vi "Main Scratch Module.vi"(8 "error in (no error)":errorcluster, 11 "main ref":T1) -> (0 "error out":errorcluster)   [LabVIEW 2025]
uses:
  controls/LAB-IQ UI Data.ctl
  Traction Loop/Traction Receipe Enum.ctl
  Scratch Main Enum.ctl
  HEAVE vi's/Heave Write enum.ctl
  b016255a-5e45-488d-a19e-9ca17f1d2554.vi
  230b88c4-d326-49ea-ab42-a573b91a982d.vi
  e59e0919-8fad-4c7c-b2ce-8f9a2e4ae2bd.vi
panel:
  out "Scratch Start Recording":bool
  out "Multi Pass Count":dbl
  out "Multi Scratch with offset":bool
  out "Distance Moved unload":dbl
  out "PID Unload Temp":bool
  out "Scratch Backward Temp":bool
  out "Distance Moved Backward":dbl
  out "Distance Moved":dbl
  out "Scratch Forward Temp":bool
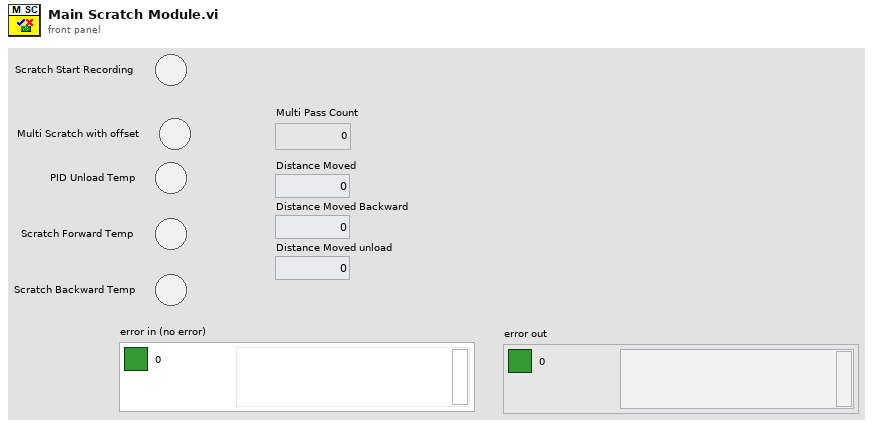
[diagram p1: front panel]
types:
  T1 = typedef "LAB-IQ UI Data.ctl" = cluster{"Main Home Screen":cluster{"GUI":refnum<vi>, "Platform Settings":refnum<vi>, "Configure":refnum<vi>, "Home":refnum<vi>, "EXIT":refnum<vi>, "service 2":refnum<vi>, "MainPage":refnum<vi>, "Analysis":refnum<vi>}, "Platform Settings":cluster{"mm/s  Surge":refnum<vi>, "Update Surge Speed":refnum<vi>, "Drive Error":refnum<vi>, "Disable Axis Jog Soft Limits":refnum<vi>, "mm/s  Sway":refnum<vi>, "Sway and Surge COM Status":refnum<vi>, "Heave COM Status":refnum<vi>, "Enable Platform":refnum<vi>, "Surge Forward Main":refnum<vi>, "Sway Right Main":refnum<vi>, "Sway Left Main":refnum<vi>, "Heave Down Main":refnum<vi>, "Heave Up main":refnum<vi>, "Update Sway Speed":refnum<vi>, "Update Heave Speed":refnum<vi>, "mm/s Heave":refnum<vi>, "mm/sec":refnum<vi>, "mm":refnum<vi>, "Surge Backward Main":refnum<vi>}, "Analysis Screen":cluster{"Analysis Home":refnum<vi>, "Surface Analysis":refnum<vi>, "Imaging":refnum<vi>, "Image Analysis":refnum<vi>, "Post Analysis":refnum<vi>}, "Config Screen":cluster{"Select Load Head":refnum<vi>, "Notes :":refnum<vi>, "FILE":refnum<vi>, "Sample ID :":refnum<vi>, "Operator ID :":refnum<vi>, "Operator Name :":refnum<vi>, "Auto":refnum<vi>}, "Motion Module":cluster{"zNL":refnum<vi>, "NL disp":refnum<vi>, "Rotary Tab":refnum<vi>, "Motion Direction:  3":refnum<vi>, "E.Velocity 2":refnum<vi>, "e.v/ssr 2":refnum<vi>, "Enter Fixed E.Velocity 2":refnum<vi>, "Enter Final SRR 2":refnum<vi>, "Enter initial SRR 2":refnum<vi>, "Enter Fixed SRR 2":refnum<vi>, "Enter the Final E.Velocity (m/s) 2":refnum<vi>, "Enter initial E.Velocity (m/s) 2":refnum<vi>, "Final Speed (RPM) 3":refnum<vi>, "Initial Speed (RPM) 2":refnum<vi>, "Enter the Final Velocity (m/s) 3":refnum<vi>, "Enter initial Velocity (m/s)  3":refnum<vi>, "Ramp Up 2":refnum<vi>, "TEST SELECTION":refnum<vi>, "SPEED SELECTION : ":refnum<vi>, "Angular Oscillation Set":refnum<vi>, "Traction":refnum<vi>, "Step Speed":refnum<vi>, "StepTable For Load-Speed":refnum<vi>, "StepTable For Speed":refnum<vi>, "Surge Forward MM":refnum<vi>, "Surge Backward MM":refnum<vi>, "M3 Image":refnum<vi>, "String 39":refnum<vi>, "Sway Left MM":refnum<vi>, "Sway Right MM":refnum<vi>, "Disable Axis Jog Soft Limits":refnum<vi>, "mm":refnum<vi>, "Heave Down MM":refnum<vi>, "Heave Up MM":refnum<vi>, "Wear Track Diameter (mm)":refnum<vi>, "Set WTD":refnum<vi>, "HomeScratch":refnum<vi>, "HomeRot":refnum<vi>, "PlaceModule":refnum<vi>, "Enter the Angle (Deg)":refnum<vi>, "Enter the Frequency (Hz)":refnum<vi>, "Motion Mode:":refnum<vi>, "LR Sway":refnum<vi>, "Rot Hor":refnum<vi>, "Scratch":refnum<vi>, "LR Cam":refnum<vi>, "MMBack":refnum<vi>, "MMNext":refnum<vi>, "Rot Ver":refnum<vi>, "Rotary Module Selection":refnum<vi>, "calculate rotary":refnum<vi>, "SPEED SELECTION : rotary":refnum<vi>, "Import 2":refnum<vi>, "Save 2":refnum<vi>, "File Path :  2":refnum<vi>, "String 45":refnum<vi>, "StepTable For Speed 3":refnum<vi>, "Enter the Speed(mm/sec)":refnum<vi>, "Enter the Speed(RPM)":refnum<vi>, "Enter Scratch Speed (mm/s):":refnum<vi>, "SwaySpeed Set":refnum<vi>, "Scartch Offset":refnum<vi>, "Motion type:":refnum<vi>, "HomeScratch 2":refnum<vi>, "Enter Scratch length (mm):":refnum<vi>, "Wear Track Diameter":refnum<vi>, "Rotary Speed Exced":refnum<vi>, "Scratch Mode":refnum<vi>, "No of Scratch":refnum<vi>}, "Environmental control":cluster{"Humidity  Status  3":refnum<vi>, "Low Temp  Status  2":refnum<vi>, "TK4 status 2":refnum<vi>, "Stage Temperature":refnum<vi>, "Sample Temperature":refnum<vi>, "Humidity (Amb)":refnum<vi>, "Clear List":refnum<vi>, "Add to list":refnum<vi>, "Wear":refnum<vi>, "Vibration":refnum<vi>, "Humidity (Chamber)":refnum<vi>, "Temperature (Chamber)":refnum<vi>, "ECR ":refnum<vi>, "Temperature (Amb)":refnum<vi>, "Microphone":refnum<vi>, "Acoustic Emission 3":refnum<vi>, "SNext":refnum<vi>, "APBack":refnum<vi>, "Enter the Temperature (°C):":refnum<vi>, "Enter the Stage \nTemperature (°C):":refnum<vi>, "Enter the Humidity (%Rh):":refnum<vi>, "Low Temp":refnum<vi>, "High Temp":refnum<vi>, "Humidity":refnum<vi>, "Sensors Picked":refnum<vi>}, "About Screen":cluster{"Password":refnum<vi>, "Home Service":refnum<vi>, "Advanced Setting":refnum<vi>, "About Tab":refnum<vi>, "ECR Port:":refnum<vi>, "Ramp Port:":refnum<vi>, "Installation/Replacement completed":refnum<vi>, "Loahead":refnum<vi>, "Heave and Surge COM Port:":refnum<vi>, "Sway COM Port:":refnum<vi>, "Temp Modbus:":refnum<vi>, "Humidity Port:":refnum<vi>, "Edit Gain Constants":refnum<vi>, "Save Gain Constants":refnum<vi>}, "Main Screen":cluster{"Main Screen Tab":refnum<vi>, "Angle and Frequency":refnum<vi>, "Stroke (mm)":refnum<vi>, "Angle (Deg)":refnum<vi>, "Main Speed Tab":refnum<vi>, "MTM MOTOR DISPLAY":refnum<vi>, "Disc Speed (m/sec)":refnum<vi>, "Ball Speed (m/sec)":refnum<vi>, "Disc Speed (RPM)":refnum<vi>, "Ball Speed (RPM)":refnum<vi>, "SPEED TAB":refnum<vi>, "Speed (m/sec)":refnum<vi>, "Set Speed (m/sec)":refnum<vi>, "Speed (RPM)":refnum<vi>, "Set Speed":refnum<vi>, "Time Tab":refnum<vi>, "Time ( HH:MM:SS ) 2":refnum<vi>, "Test Duration":refnum<vi>, "Test Duration 4":refnum<vi>, "TEST CYCLE":refnum<vi>, "TOTAL CYCLES":refnum<vi>, "Set Load (N)":refnum<vi>, "Temp Tabs":refnum<vi>, "Heater":refnum<vi>, "TK4 status":refnum<vi>, "ChamberTemp":refnum<vi>, "SetTmp":refnum<vi>, "Controller  Status":refnum<vi>, "ChamberTemp 2":refnum<vi>, "SetTmp 2":refnum<vi>, "Controller  Status 2":refnum<vi>, "ChamberTemp 3":refnum<vi>, "SetTmp 3":refnum<vi>, "Cooling":refnum<vi>, "Load Communication":refnum<vi>, "Ambient \nTemperature":refnum<vi>, "HumCOMStatus":refnum<vi>, "Ambient\n Humidity":refnum<vi>, "Freq (Hz)":refnum<vi>, "Load En":refnum<vi>, "NLt":refnum<vi>, "zNL 2":refnum<vi>, "Humidity On":refnum<vi>, "humidity disp":refnum<vi>, "Set Humidity":refnum<vi>, "NL disp 2":refnum<vi>, "Humidity On 2":refnum<vi>, "humidity disp 2":refnum<vi>, "Set Humidity 2":refnum<vi>, "NL disp 3":refnum<vi>, "AppLoadSeq scratch":refnum<vi>, "Stop Scratch":refnum<vi>, "ClrLog":refnum<vi>, "Trip Log":refnum<vi>, "STOP":refnum<vi>, "Start Test":refnum<vi>, "Test status":refnum<vi>, "AR Led":refnum<vi>, "Data":refnum<vi>, "Health":refnum<vi>, "Sway COM Status":refnum<vi>, "Heave COM Status":refnum<vi>, "Grp Tab":refnum<vi>, "Sub Graph":refnum<vi>, "SD (mm)":refnum<vi>, "Siliding distance Reset Graph":refnum<vi>, "SDGp":refnum<vi>, "Humidity Reset Graph":refnum<vi>, "HumrGp":refnum<vi>, "Acoustic Emission (mV)":refnum<vi>, "Aqucostic Reset Graph":refnum<vi>, "gACQUOS":refnum<vi>, "ECR RESET":refnum<vi>, "ECR":refnum<vi>, "Temperature Reset":refnum<vi>, "Acoustic Emission (mV) 2":refnum<vi>, "Aqucostic Reset Graph 2":refnum<vi>, "gACQUOS 2":refnum<vi>, "ECR RESET 2":refnum<vi>, "ECR 2":refnum<vi>, "Temperature Reset 2":refnum<vi>, "Temperature (deg c)":refnum<vi>, "Speed Reset Graph":refnum<vi>, "Speed Tab":refnum<vi>, "MTM DISC  SPEED":refnum<vi>, "MTM BALL SPEED":refnum<vi>, "speed mm/sec":refnum<vi>, "Hymidity":refnum<vi>, "Humidity Disable trip":refnum<vi>, "CoF Trip  2":refnum<vi>, "Depth Trip":refnum<vi>, "Weart Deapth":refnum<vi>, "Depth Reset Graph":refnum<vi>, "Weart":refnum<vi>, "Depthz":refnum<vi>, "Depth (µm)":refnum<vi>, "WearGp":refnum<vi>, "NL Trip 2":refnum<vi>, "Load pid":refnum<vi>, "Load Disable Trip":refnum<vi>, "Load Reset Graph":refnum<vi>, "NL Display 4":refnum<vi>, "Main Chart 3":refnum<vi>, "BACK":refnum<vi>, "Depth Trip 2":refnum<vi>, "COF TRIP ":refnum<vi>, "Friction Force (N)":refnum<vi>, "FF Reset Graph":refnum<vi>, "FF Disable Trip":refnum<vi>, "FF TRIP":refnum<vi>, "COF Disable Trip":refnum<vi>, "COF Reset Graph":refnum<vi>, "Start Test Temp":refnum<vi>, "zFF":refnum<vi>, "Friction Force (N) Graph":refnum<vi>, "Coefficient of Friction":refnum<vi>, "Scratch Start Test":refnum<vi>, "FF Tab":refnum<vi>, "Cyclic Friction Force (N)":refnum<vi>, "CZ FF":refnum<vi>, "Cyclic Friction Force (N) Graph":refnum<vi>, "Cyclic Coefficient of Friction":refnum<vi>, "Cyclic FF TRIP":refnum<vi>, "Cyclic FF Disable Trip":refnum<vi>, "cyclic COF Disable Trip":refnum<vi>, "cyclic COF TRIP":refnum<vi>, "cyclic COF Reset Graph":refnum<vi>, "Cyclic FF Reset Graph":refnum<vi>, "Test Trip":refnum<vi>, "Multi Scratch Pass":refnum<vi>, "Scratch Start Recording":refnum<vi>}, "Loading":cluster{"Indentation":refnum<vi>, "Reference Sample":refnum<vi>, "Load Cell Communication Slide":refnum<vi>, "com 3":refnum<vi>, "com":refnum<vi>, "DecaForce COM Status":refnum<vi>, "Update":refnum<vi>, "Clear 3":refnum<vi>, "seq":refnum<vi>, "Stribeck table":refnum<vi>, "Stribeck Table  For loading":refnum<vi>, "Loading Mode":refnum<vi>, "Enter the Final Load (N)":refnum<vi>, "Enter the CoF Trip":refnum<vi>, "Enter the Friction Force Trip":refnum<vi>, "Enter the Normal load Trip":refnum<vi>, "Enter the Load  (N)":refnum<vi>, "KiloForce":refnum<vi>, "DecaForce ":refnum<vi>, "MicroForce":refnum<vi>, "LHBack":refnum<vi>, "LHNext":refnum<vi>, "Enter the Loading Rate (N/min)":refnum<vi>, "Message":refnum<vi>, "Warning 2":refnum<vi>, "SSP 0.75":refnum<vi>, "SSP 0.5":refnum<vi>, "SSP 0.3":refnum<vi>, "Warning":refnum<vi>, "gui GIF":refnum<vi>, "Communication is established":refnum<vi>, "AppLoad 4":refnum<vi>, "Multipoint":refnum<vi>, "Load Selection":refnum<vi>}, "PID":cluster{"Ramp MulFac":refnum<vi>, "pulses LoadDiffRamp(2..10)":refnum<vi>, "PulseControlRamp(diff<=3N)":refnum<vi>, "SetLoadDeadband(%) Load(0-10N)":refnum<vi>, "PID gains out delay (microForce)":refnum<vi>, "Ramp":refnum<vi>, "Gain 2":refnum<vi>, "pulses LoadDiff(2..10)":refnum<vi>, "pulses LoadDiff(11..50)":refnum<vi>, "PulseControl(diff<=3N)":refnum<vi>, "SetLoadDeadband(%)  2":refnum<vi>, "Dummy Run":refnum<vi>, "Vertical load (N)":refnum<vi>, "AutoTune":refnum<vi>, "Offset 3 ":refnum<vi>, "apply load":refnum<vi>, "Offset  3":refnum<vi>, "apply load 2":refnum<vi>, "Enter ByPass Load":refnum<vi>, "reinit 3":refnum<vi>, "output range delay":refnum<vi>, "PID gains out delay":refnum<vi>, "Bypass Load":refnum<vi>, "pulsesSent":refnum<vi>, "pulses ":refnum<vi>, "actpid":refnum<vi>, "gFF Rot":refnum<vi>, "pulses LoadDiff(21..1000)":refnum<vi>, "Delay":refnum<vi>, "deadband":refnum<vi>}, "Config Parameters":cluster{"Tab Control 3":refnum<vi>, "Tab Control 19":refnum<vi>, "SAMPLES":refnum<vi>, "Re-initilaize":refnum<vi>, "Filter ON/OFF":refnum<vi>, "TracHomeSurgeOffsetCounts 10MM":refnum<vi>, "TracHomeSwayOffsetCounts 10MM":refnum<vi>, "Acoustic Emission:":refnum<vi>, "Apply Filter (FF)":refnum<vi>, "Filter% 2":refnum<vi>, "Apply Filter (Load)":refnum<vi>, "Filter% ":refnum<vi>, "Sway distance (mm)":refnum<vi>, "Surge distance (mm)":refnum<vi>, "DataSavingLoopDelay(ms)":refnum<vi>, "SAVE 2":refnum<vi>, "Enter Distance":refnum<vi>, "Sway Counts:":refnum<vi>, "Distance (mm): 3":refnum<vi>, "Surge Counts:":refnum<vi>, "Distance (mm): 2":refnum<vi>, "Distance (mm):":refnum<vi>, "Heave Counts:":refnum<vi>, "LRMHomeSurgeOffsetCounts":refnum<vi>, "LRMHomeSwayOffsetCounts":refnum<vi>, "TracHomeSurgeOffsetCounts 20MM":refnum<vi>, "TracHomeSwayOffsetCounts 20MM":refnum<vi>, "RotHomeSwayOffsetCounts":refnum<vi>, "RotHomeSurgeOffsetCounts":refnum<vi>, "Heave distance":refnum<vi>, "Zmm":refnum<vi>, "Heave Pulses/mm":refnum<vi>, "Surge Pulses/mm":refnum<vi>, "Sway Pulses/mm":refnum<vi>, "Heave Pitch":refnum<vi>, "Surge Pitch":refnum<vi>, "Sway Pitch":refnum<vi>, "Heave PPR":refnum<vi>, "Surge PPR":refnum<vi>, "Sway PPR":refnum<vi>, "Tab Control 5":refnum<vi>, "Tab Control 14":refnum<vi>, "Tab Control 26":refnum<vi>, "AE":refnum<vi>, "Heave Loop Delay":refnum<vi>, "Heave PID Speed":refnum<vi>, "Surge Jog Speed":refnum<vi>, "Heave Jog Speed":refnum<vi>, "Sway Loop Delay":refnum<vi>, "Sway PID Speed":refnum<vi>, "Sway Jog Speed":refnum<vi>, "DEPTH TRIP VALUE":refnum<vi>, "LOAD TRIP VALUE":refnum<vi>, "DEPTH TRIP   ENABLE":refnum<vi>, "LOAD TRIP  ENABLE":refnum<vi>, "CYCLIC FF TRIP VALUE":refnum<vi>, "FF TRIP VALUE":refnum<vi>, "CYCLIC CoF TRIP VALUE":refnum<vi>, "COF TRIP VALUE":refnum<vi>, "CYCLIC COF TRIP  ENABLE":refnum<vi>, "CYCLIC FF TRIP  ENABLE":refnum<vi>, "FF TRIP  ENABLE":refnum<vi>, "COF TRIP  ENABLE":refnum<vi>, "JOG TRIP LOAD VALUE (N)":refnum<vi>, "Rotary Vertical":refnum<vi>, "Traction":refnum<vi>, "Scratch":refnum<vi>, "LRM CAM":refnum<vi>, "Sway LRM":refnum<vi>, "Rotary Horizontal":refnum<vi>}, "Loading Com Port":cluster{"ClearAll":refnum<vi>, "Mz(Nm)":refnum<vi>, "My(Nm)":refnum<vi>, "Mx(Nm)":refnum<vi>, "Save Dwell":refnum<vi>, "Acq Delay (ms)":refnum<vi>, "Burst Delay (ms)":refnum<vi>, "model":refnum<vi>, "SN":refnum<vi>, "FFx(N)":refnum<vi>, "Sensor IP":refnum<vi>, "Port":refnum<vi>, "FFy(N)":refnum<vi>, "Load(N)":refnum<vi>, "delete Handle":refnum<vi>, "Create Handle":refnum<vi>, "ft_data":refnum<vi>, "ft_range":refnum<vi>, "ft_data 2":refnum<vi>, "stop 6":refnum<vi>, "running_flag":refnum<vi>, "ft_udp_handle":refnum<vi>, "get-data-return":refnum<vi>, "get-range-return":refnum<vi>, "zero-return":refnum<vi>, "filter-return":refnum<vi>, "initial-return":refnum<vi>, "deleteHandle-result":refnum<vi>, "Load Cell Temp":refnum<vi>, "Load Cell":refnum<vi>, "ZeroAll":refnum<vi>, "FORCE (N)":refnum<vi>, "TORQUE (N-m)":refnum<vi>}, "Heave AND Surge":cluster{"SURGE POSE":refnum<vi>, "error out Read":refnum<vi>, "HEAVE POSE":refnum<vi>, "State":refnum<vi>, "Homed":refnum<vi>, "Sequence ID":refnum<vi>, "error out Write":refnum<vi>, "faultCode":refnum<vi>, "Ack ID":refnum<vi>, "SPEED":refnum<vi>, "Distance":refnum<vi>, "Mode Command":refnum<vi>, "Heave and Surge Read":refnum<vi>, "Read Heave Temp":refnum<vi>, "Spare 15":refnum<vi>, "Spare 14":refnum<vi>, "Spare 13":refnum<vi>, "Spare 12":refnum<vi>, "Spare 11":refnum<vi>, "Spare 10":refnum<vi>, "Spare 9":refnum<vi>, "Spare 8":refnum<vi>, "Spare 7":refnum<vi>, "Spare 6":refnum<vi>, "Spare 5":refnum<vi>, "Spare 4":refnum<vi>, "Spare 2":refnum<vi>, "Spare 1":refnum<vi>, "Node Id":refnum<vi>, "Spare 3":refnum<vi>, "SPARE 4":refnum<vi>, "SPARE 3":refnum<vi>, "SPARE 2":refnum<vi>, "SPARE 1":refnum<vi>, "fwMajor":refnum<vi>, "fwMinor":refnum<vi>, "Manual Write":refnum<vi>, "Heave and Surge Write":refnum<vi>, "SPARE 5":refnum<vi>, "Reserved ":refnum<vi>, "SPARE 8":refnum<vi>, "SPARE 6":refnum<vi>, "SPARE 7":refnum<vi>, "SPARE 17":refnum<vi>, "SPARE 16":refnum<vi>, "SPARE 15":refnum<vi>, "SPARE 14":refnum<vi>, "SPARE 13":refnum<vi>, "SPARE 12":refnum<vi>, "SPARE 11":refnum<vi>, "SPARE 10":refnum<vi>, "SPARE 9":refnum<vi>, "System UPTIME":refnum<vi>, "Missed Packets":refnum<vi>, "faultCode Surge Right":refnum<vi>, "faultCode Surge Left":refnum<vi>, "faultCode Heave":refnum<vi>, "UPLINK HEAVE":refnum<vi>, "DOWNLINK HEAVE":refnum<vi>}, "New PID LOGIC":cluster{"Fine Tune Zone":refnum<vi>, "PID SDelay":refnum<vi>, "Max_pos_limit":refnum<vi>, "Min_pos_limit":refnum<vi>, "i_limit":refnum<vi>, "pct_scale":refnum<vi>, "Deadband":refnum<vi>, "Kd":refnum<vi>, "Ki":refnum<vi>, "Kp":refnum<vi>, "Current Position":refnum<vi>, "Set Load":refnum<vi>, "Current Load":refnum<vi>, "Pulse delta":refnum<vi>, "Init Step":refnum<vi>, "Max Step Linit":refnum<vi>, "min_deadband_floor":refnum<vi>, "dynamic_spindle_noise_scalar":refnum<vi>, "min_finetune_floor":refnum<vi>, "filter_alpha":refnum<vi>, "PID":refnum<vi>}, "SWAY ":cluster{"fwMajor":refnum<vi>, "Homed":refnum<vi>, "Rotary POSE":refnum<vi>, "State":refnum<vi>, "SWAY POSE":refnum<vi>, "Ack ID":refnum<vi>, "faultCode":refnum<vi>, "Node Id":refnum<vi>, "fwMinor":refnum<vi>, "Spare 6":refnum<vi>, "Spare 5":refnum<vi>, "Spare 4":refnum<vi>, "Spare 3":refnum<vi>, "Spare 2":refnum<vi>, "Spare 1":refnum<vi>, "Spare 7":refnum<vi>, "SPARE  5":refnum<vi>, "error out Write  SWAY ":refnum<vi>, "error out Read SWAY ":refnum<vi>, "Manual Write SWAY ":refnum<vi>, "SWAY WRITE":refnum<vi>, "SPARE  4":refnum<vi>, "SPARE  3":refnum<vi>, "SPARE 2":refnum<vi>, "SPARE 1":refnum<vi>, "Spare 15":refnum<vi>, "Spare 14":refnum<vi>, "Spare 13":refnum<vi>, "Spare 12":refnum<vi>, "Spare 11":refnum<vi>, "Spare 9":refnum<vi>, "Spare 8":refnum<vi>, "SPEED":refnum<vi>, "Distance":refnum<vi>, "Mode Command":refnum<vi>, "Sequence ID":refnum<vi>, "SWAY READ":refnum<vi>, "Spare 10":refnum<vi>, "Read SWAY Temp":refnum<vi>, "faultCode Sway ":refnum<vi>, "Missed Packets":refnum<vi>, "System UPTIME sway":refnum<vi>, "SPARE 6":refnum<vi>, "SPARE 7":refnum<vi>, "SPARE 9":refnum<vi>, "SPARE 11":refnum<vi>, "SPARE 10":refnum<vi>, "SPARE 8":refnum<vi>, "SPARE 13":refnum<vi>, "SPARE 12":refnum<vi>, "SPARE 17":refnum<vi>, "SPARE 16":refnum<vi>, "SPARE 15":refnum<vi>, "SPARE 14":refnum<vi>, "Reserved":refnum<vi>, "faultCode Rotary":refnum<vi>, "UPLINK SWAY":refnum<vi>, "DOWNLINK SWAY":refnum<vi>}, "Analysis Screen":cluster{"Analysis Home":refnum<vi>, "Refresh 2":refnum<vi>, "MEAN 4":refnum<vi>, "SD 4":refnum<vi>, "VARIANCE 4":refnum<vi>, "MEAN  3":refnum<vi>, "SD  3":refnum<vi>, "VARIANCE  3":refnum<vi>, "MEAN 2":refnum<vi>, "SD  2":refnum<vi>, "VARIANCE 2":refnum<vi>, "MEAN":refnum<vi>, "SD":refnum<vi>, "VARIANCE":refnum<vi>, "File 4 Discription":refnum<vi>, "OPEN 4":refnum<vi>, "File Name 4":refnum<vi>, "OPEN 3":refnum<vi>, "File 3 Discription":refnum<vi>, "File Name 3":refnum<vi>, "Y-AXIS":refnum<vi>, "X-AXIS":refnum<vi>, "XY Graph":refnum<vi>, "File Name 2":refnum<vi>, "File Name 1":refnum<vi>, "OPEN 2":refnum<vi>, "OPEN 1":refnum<vi>, "File 1 Discription ":refnum<vi>, "File 2 Discription":refnum<vi>, "Export":refnum<vi>, "File Format":refnum<vi>}, "Traction":cluster{"faultCode Traction 2":refnum<vi>, "faultCode Traction 1":refnum<vi>, "Missed Packets":refnum<vi>, "System UPTIME Traction":refnum<vi>, "SPARE 17":refnum<vi>, "SPARE 16":refnum<vi>, "SPARE 15":refnum<vi>, "SPARE 14":refnum<vi>, "SPARE 13":refnum<vi>, "SPARE 12":refnum<vi>, "SPARE 11":refnum<vi>, "SPARE 10":refnum<vi>, "SPARE 9":refnum<vi>, "SPARE 8":refnum<vi>, "SPARE 7":refnum<vi>, "SPARE 6":refnum<vi>, "Reserved":refnum<vi>, "SPARE  5":refnum<vi>, "Manual Write TRACTION":refnum<vi>, "TRACTION WRITE":refnum<vi>, "SPARE  4":refnum<vi>, "SPARE  3":refnum<vi>, "SPARE 2":refnum<vi>, "SPARE 1":refnum<vi>, "Spare 7":refnum<vi>, "Spare 6":refnum<vi>, "Spare 5":refnum<vi>, "Spare 4":refnum<vi>, "Spare 2":refnum<vi>, "Spare 1":refnum<vi>, "Node Id":refnum<vi>, "Read TRACTION Temp":refnum<vi>, "fwMinor":refnum<vi>, "fwMajor":refnum<vi>, "faultCode":refnum<vi>, "TRACTION POSE":refnum<vi>, "TRACTION POSE 2":refnum<vi>, "Homed":refnum<vi>, "State":refnum<vi>, "Ack ID":refnum<vi>, "SPEED":refnum<vi>, "Distance":refnum<vi>, "Mode Command":refnum<vi>, "Sequence ID":refnum<vi>, "error out Read TRACTION":refnum<vi>, "error out Write  TRACTION":refnum<vi>, "TRACTION READ":refnum<vi>, "Spare 3":refnum<vi>, "Downlink traction":refnum<vi>, "Uplink Traction":refnum<vi>}, "Traction reciepe":cluster{"SRR Sweep Range (%) Stribeck":refnum<vi>, "Traction Receipe":refnum<vi>, "Total Execution Time":refnum<vi>, "Total Steps":refnum<vi>, "Duration / Step (s)  Stribeck":refnum<vi>, "STRIBECK Fixed SRR List (%)":refnum<vi>, "Duration / Step (s) Traction":refnum<vi>, "SRR Sweep Range (%) traction":refnum<vi>, "Rolling Speed (mm/s)":refnum<vi>, "Temperature Stages (°C)":refnum<vi>, "Ball Load (N)":refnum<vi>, "Lubricant Name":refnum<vi>, "Profile File Name":refnum<vi>, "SET entrainment Velocity":refnum<vi>, "Test Array Size":refnum<vi>, "SRR INDEX [ STRIBECK]":refnum<vi>, "Stribeck Size":refnum<vi>, "SET SRR":refnum<vi>, "ELAPSED TIMER ":refnum<vi>, "BALL SET RPM":refnum<vi>, "DISC SET RPM":refnum<vi>, "SET LOAD":refnum<vi>, "TEMPERATURE READ":refnum<vi>, "SET TEMPERATURE":refnum<vi>, "Traction Size":refnum<vi>, "DISC SPEED (rpm)":refnum<vi>, "BALL SPEED (rpm)":refnum<vi>, "BALL WEAR TRACK":refnum<vi>, "DISC WEARTRACK":refnum<vi>, "SRR INDEX [ TRACTION]":refnum<vi>, "Start Index Type":refnum<vi>, "Enum - Menu":refnum<vi>, "Ball (mm/sec)":refnum<vi>, "Disc (mm/sec)":refnum<vi>}, "Traction Control":cluster{"HomeTraction":refnum<vi>, "Demo Mode Display":refnum<vi>, "Traction Message":refnum<vi>, "Traction Step Update Details":refnum<vi>, "Main Tab sequence for selection":refnum<vi>, "Ramp Tab":refnum<vi>, "e.v/ssr":refnum<vi>, "Enter Fixed E.Velocity":refnum<vi>, "Enter Final SRR":refnum<vi>, "Enter initial SRR":refnum<vi>, "Enter Fixed SRR":refnum<vi>, "Enter the Final E.Velocity (m/s)":refnum<vi>, "Enter initial E.Velocity (m/s)":refnum<vi>, "Ball WTD":refnum<vi>, "E.Velocity":refnum<vi>, "Enter the Final Velocity (m/s)":refnum<vi>, "Enter initial Velocity (m/s)":refnum<vi>, "Ramp Up   Disc":refnum<vi>, "Initial DiscSpeed (RPM)":refnum<vi>, "Final Speed (RPM) Ball":refnum<vi>, "Final Speed (RPM)":refnum<vi>, "Initial Speed (RPM) Ball":refnum<vi>, "Enter the Final Velocity (m/s) Ball":refnum<vi>, "Enter initial Velocity (m/s) Ball":refnum<vi>, "Ramp Up":refnum<vi>, "ExceedBallSpeed step":refnum<vi>, "ExceedDiscSpeed":refnum<vi>, "BallSpeed Exceed Indication":refnum<vi>, "Apply":refnum<vi>, "SPEED SELECTION : MTM":refnum<vi>, "SPEED SELECTION : MTM 2":refnum<vi>, "TEST SELECTION (MTM)":refnum<vi>, "MTM Test Selection":refnum<vi>, "File Path Tab":refnum<vi>, "File Path String":refnum<vi>, "Save":refnum<vi>, "Save  2":refnum<vi>, "Import ":refnum<vi>, "File Path :":refnum<vi>, "Step Sequence Indication Tab":refnum<vi>, "Step Sequence Indication":refnum<vi>, "Calculate Step":refnum<vi>, "StepTable":refnum<vi>, "ExceedDiscSpeed  Cinstant Speed":refnum<vi>, "ExceedBallSpeed Constant":refnum<vi>, "TEST SELECTION (MTM) 2":refnum<vi>, "SPEED SELECTION : MTM 3":refnum<vi>, "MTM Test Selection 2":refnum<vi>, "Enter the Speed (m/sec): ":refnum<vi>, "Enter the Speed (m/sec):  2":refnum<vi>, "Enter the Speed (RPM):":refnum<vi>, "Lower Spped ":refnum<vi>, "Upper":refnum<vi>, "Enter the Speed (RPM):Ball":refnum<vi>, "Disc Motion Direction: ":refnum<vi>, "Ball Motion Direction :":refnum<vi>, "Motion Mode: ":refnum<vi>, "Wear Track Diameter (mm) ":refnum<vi>, "Disc Speed Indicator":refnum<vi>, "ExceedBallSpeed":refnum<vi>}, "Acquostic":cluster{"Last Config Rejected ":refnum<vi>, "rx command count":refnum<vi>, "Current Filter Id":refnum<vi>, "Isolated Gain":refnum<vi>, "DAQ Status":refnum<vi>, "error out":refnum<vi>, "error in (no error)":refnum<vi>, "Uplink Packet":refnum<vi>, "data out":refnum<vi>, "Downlink Packet":refnum<vi>, "Signal Energy":refnum<vi>, "Amplitude db_AE":refnum<vi>, "Peak Amplitude":refnum<vi>, "AE Ring-Down Counts":refnum<vi>, "Gains":refnum<vi>, "Manual Write Acquostic":refnum<vi>}}
  T2 = enum32{"Setup", "Load Head", "Motion Module", "Environment", "Begin"}
  T3 = typedef "Scratch Main Enum.ctl" = enum16{"Init", "Start", "Load", "Scratch Forward", "Scratch Backward", "Unload", "Offest", "Close"}
  T4 = typedef "Heave Write enum.ctl" = enum16{"INIT", "WRITE", "CLOSE", "REINIT"}
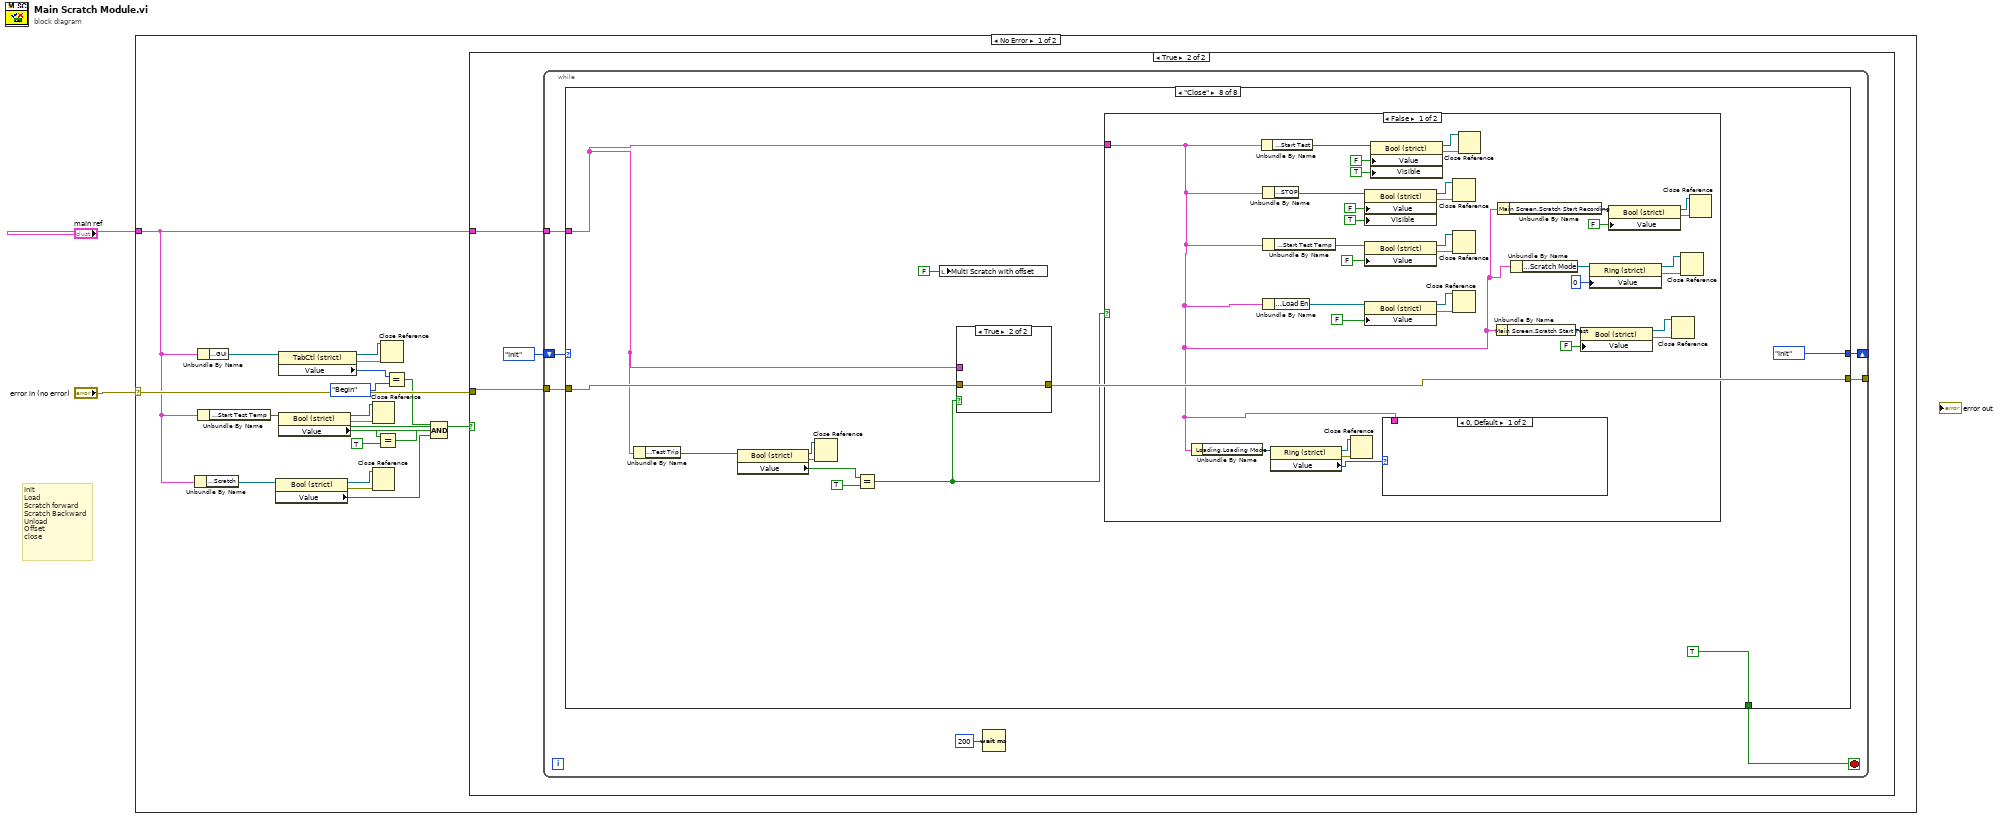
[diagram p0: block diagram]
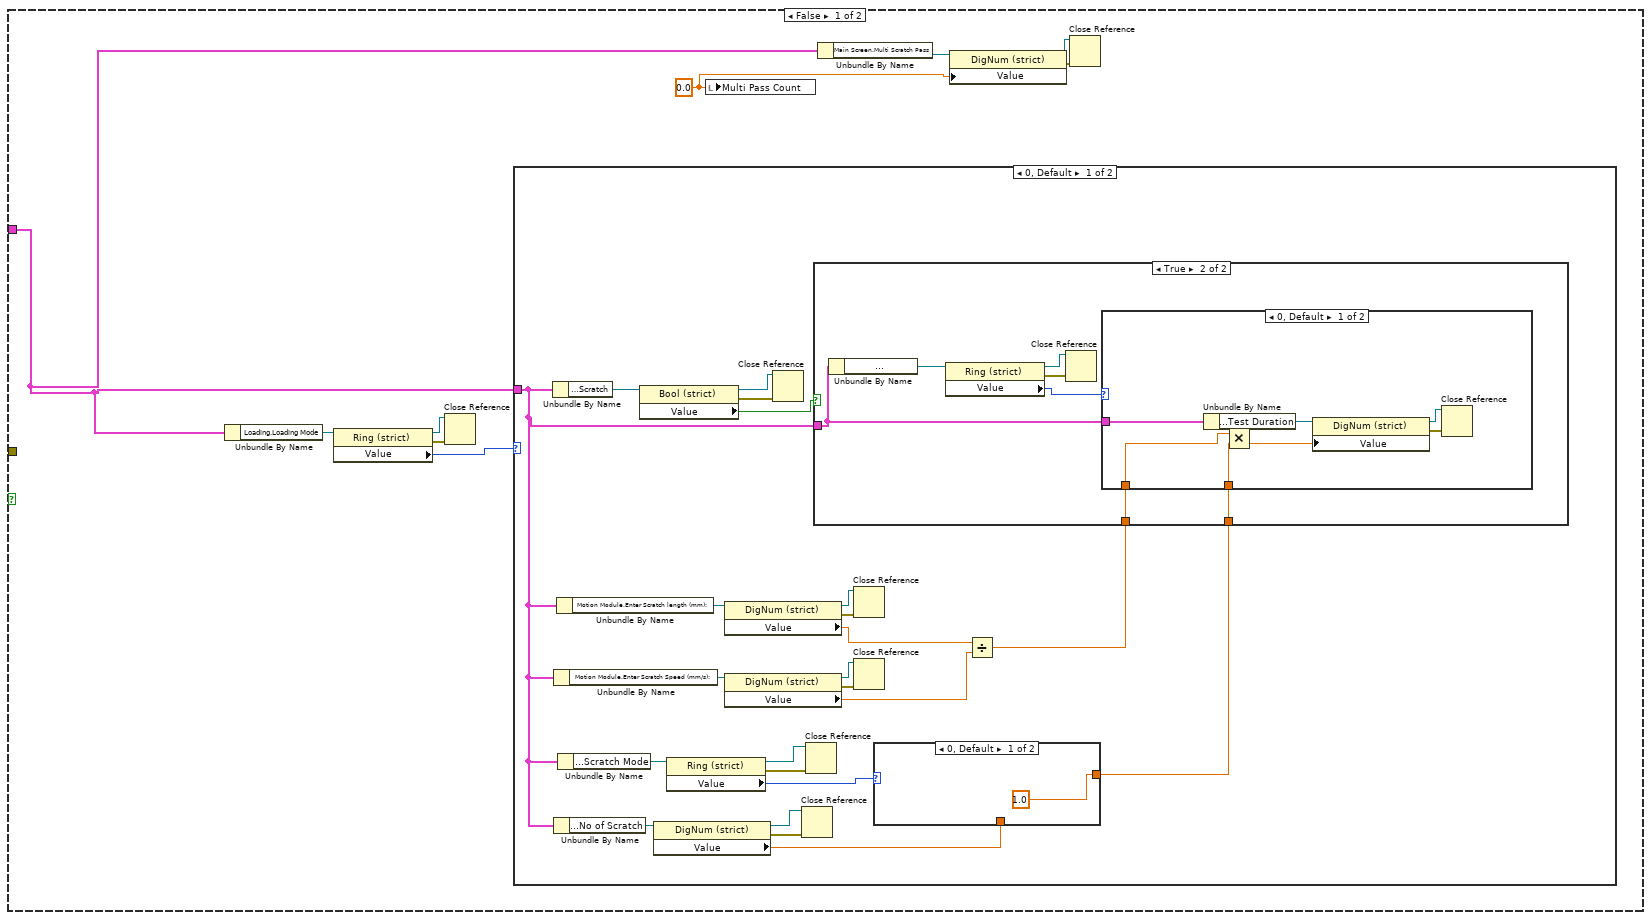
[diagram p2: hidden frame]
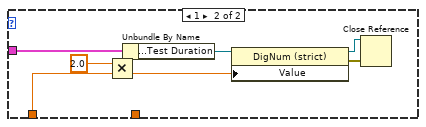
[diagram p5: hidden frame]
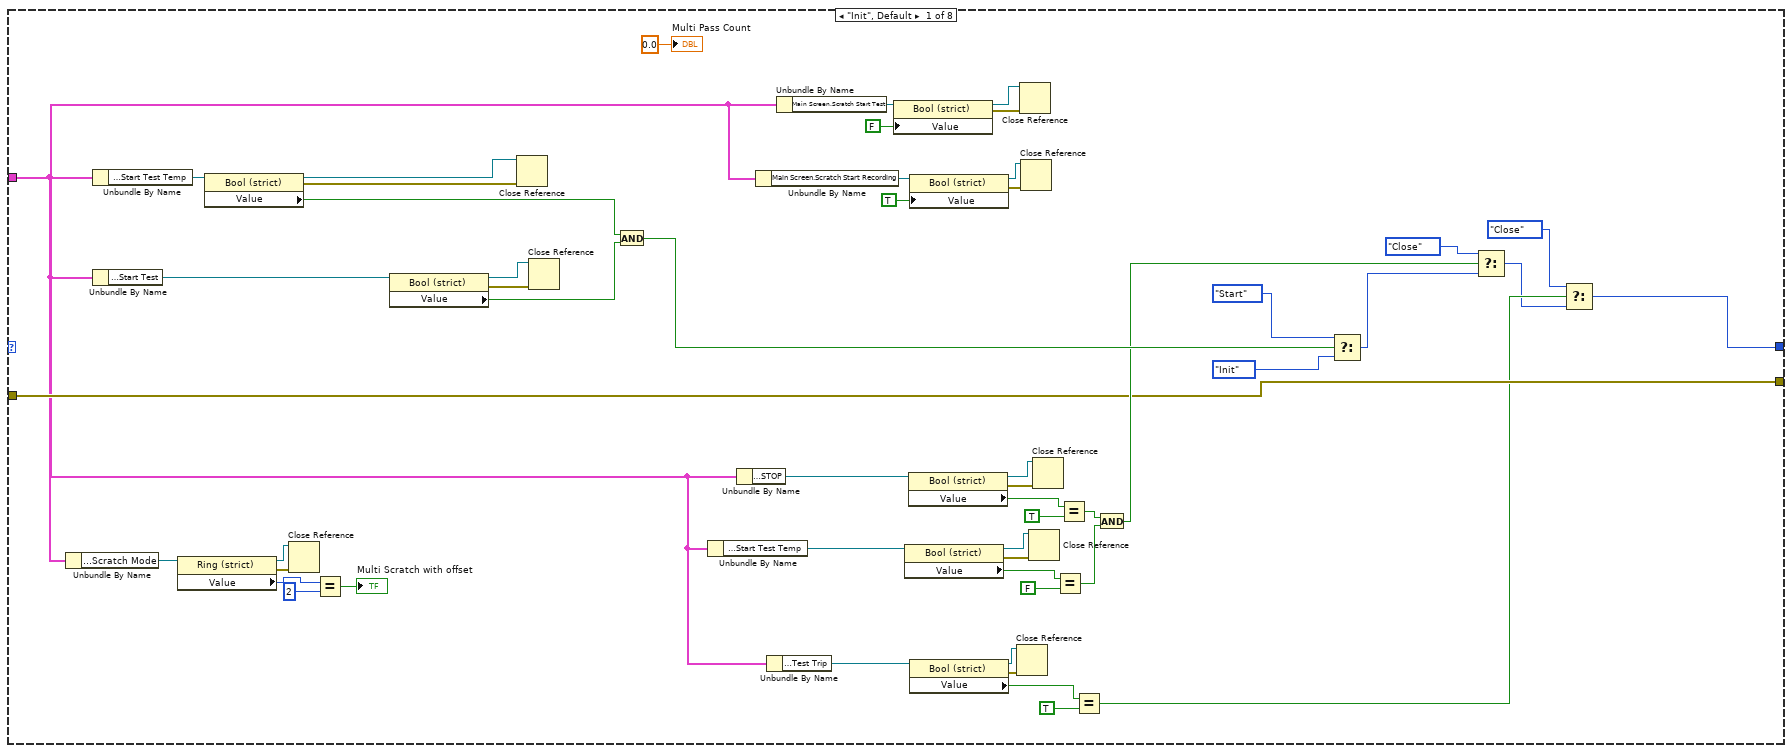
[diagram p7: hidden frame]
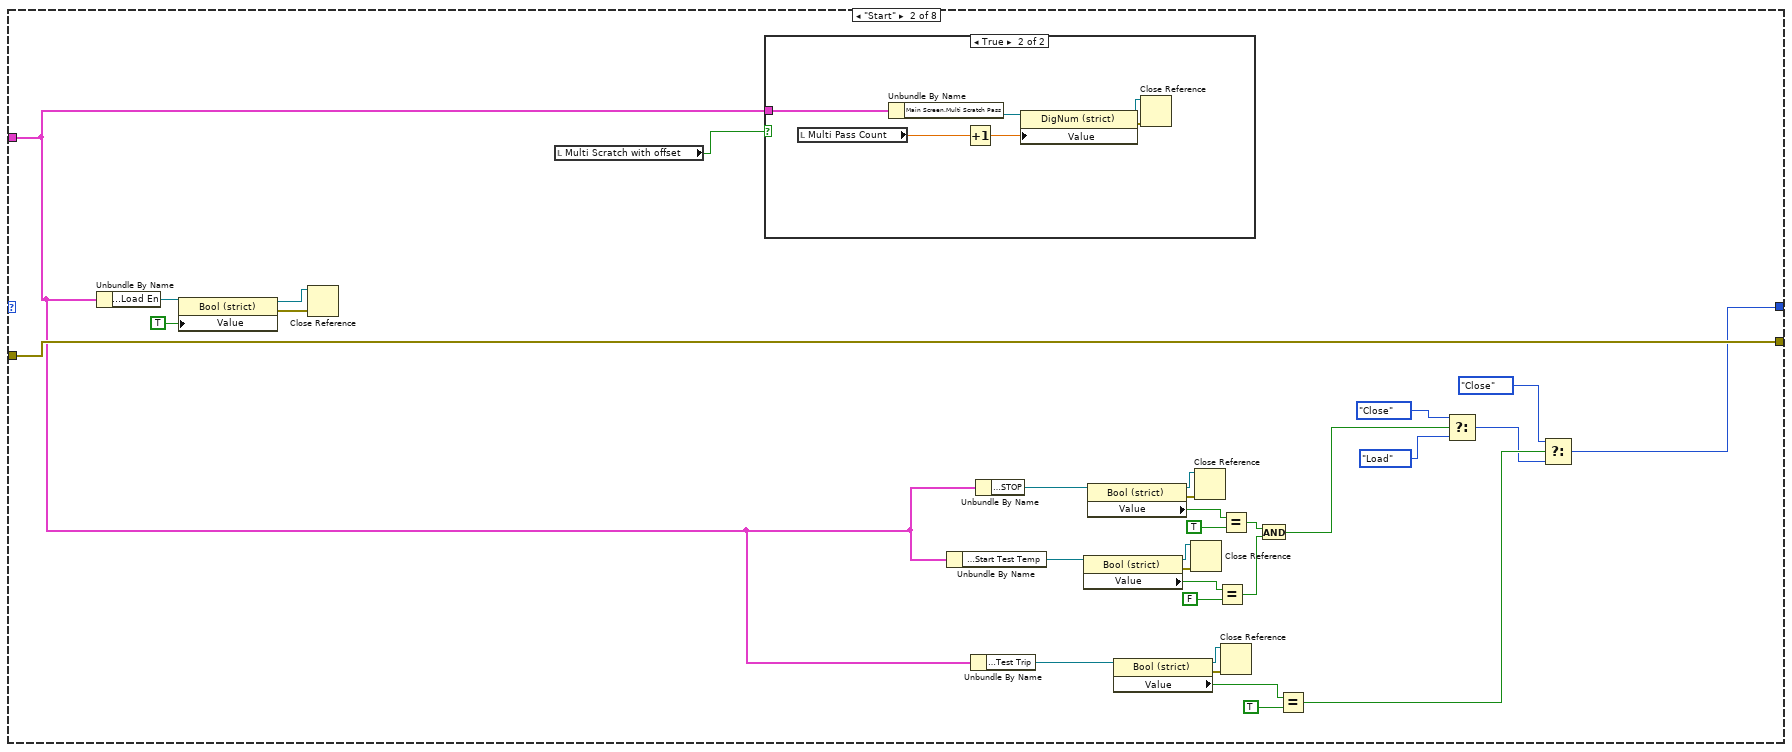
[diagram p8: hidden frame]
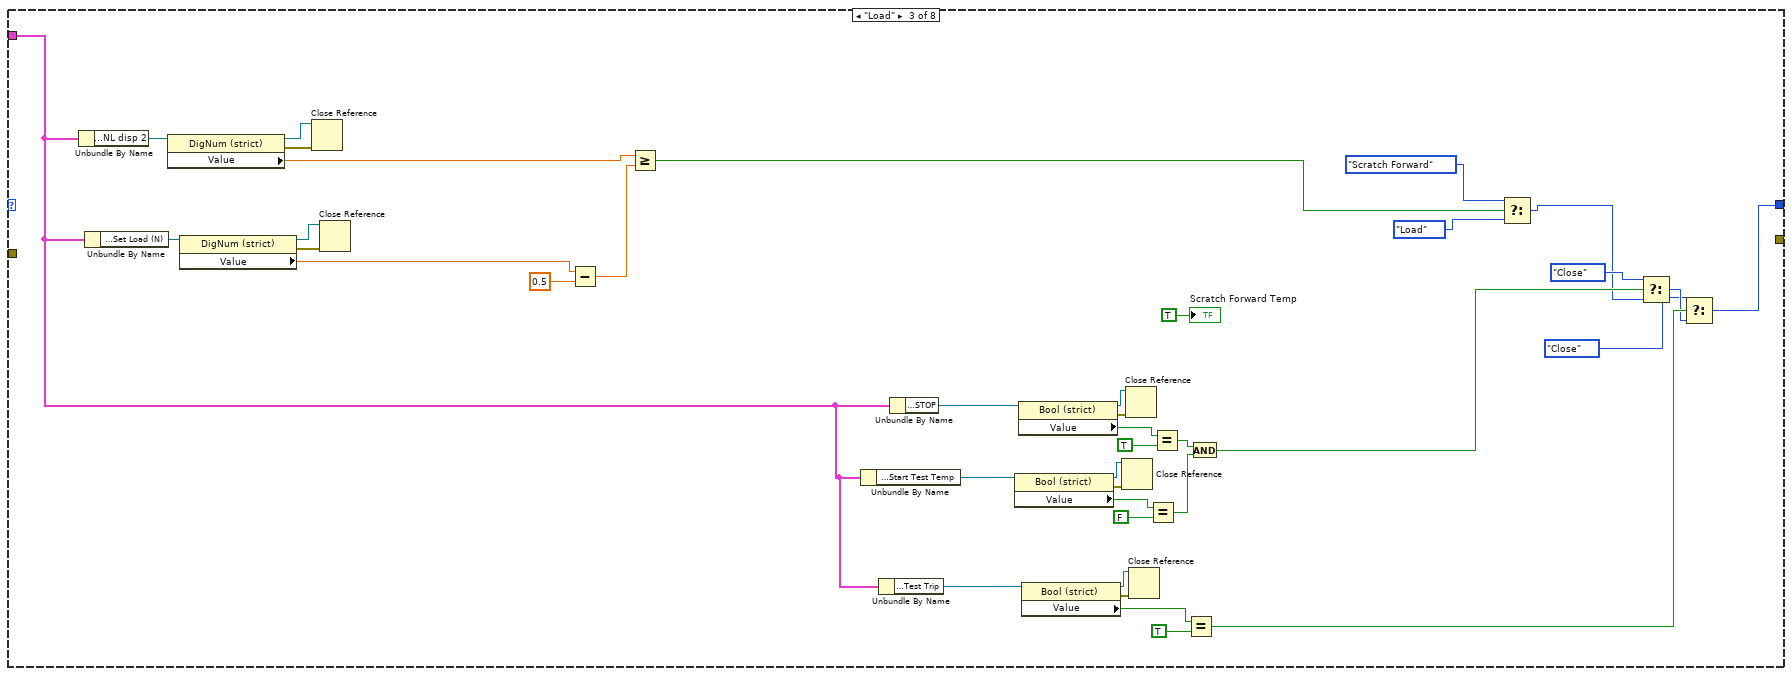
[diagram p10: hidden frame]
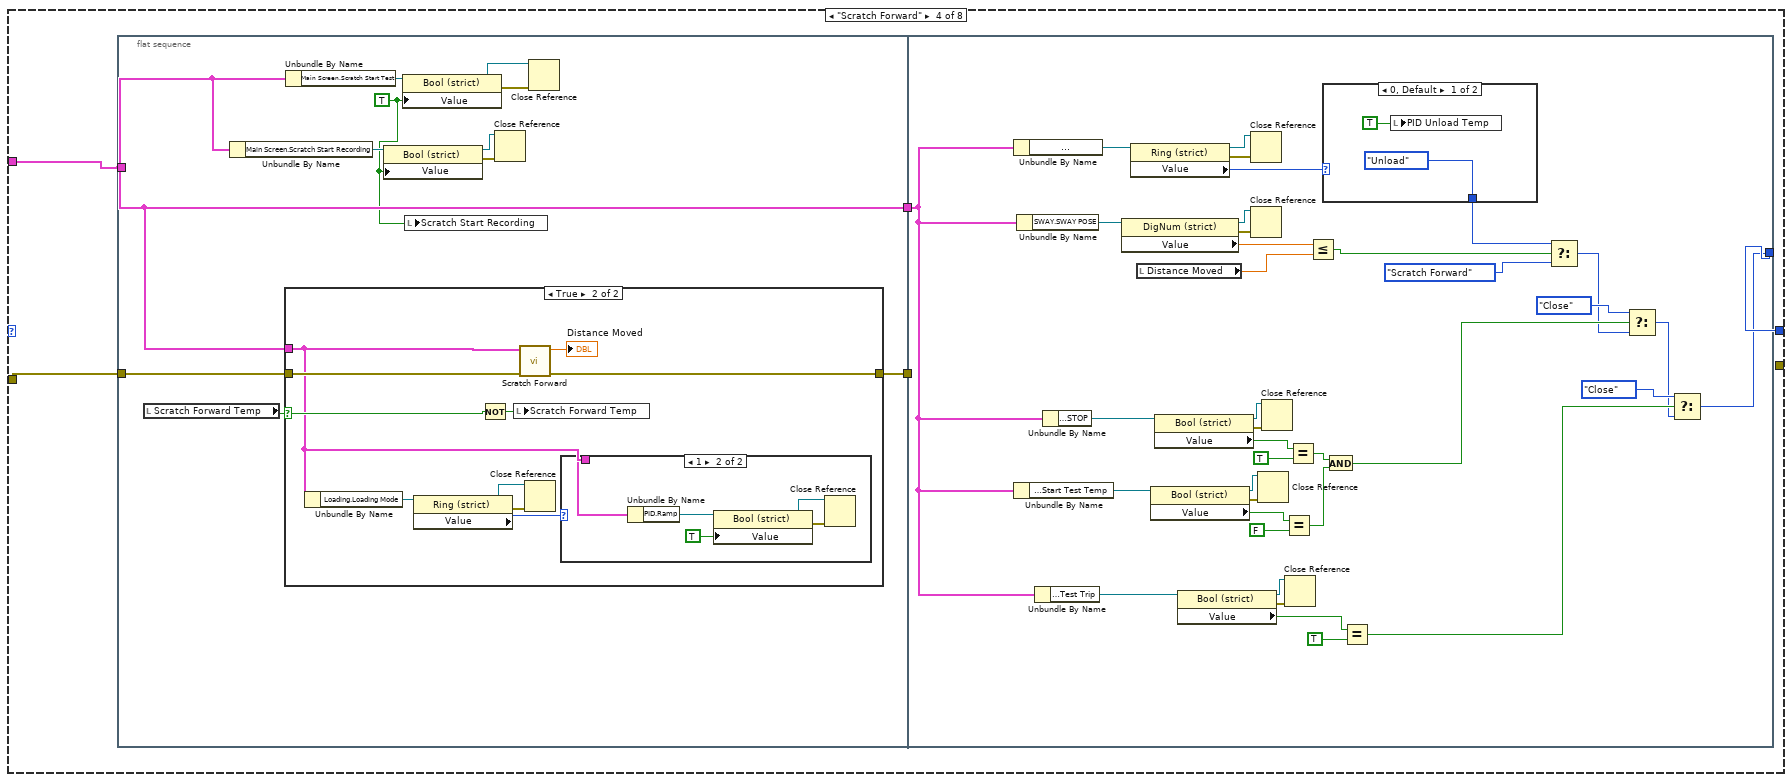
[diagram p11: hidden frame]
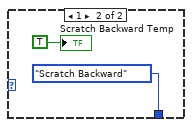
[diagram p14: hidden frame]
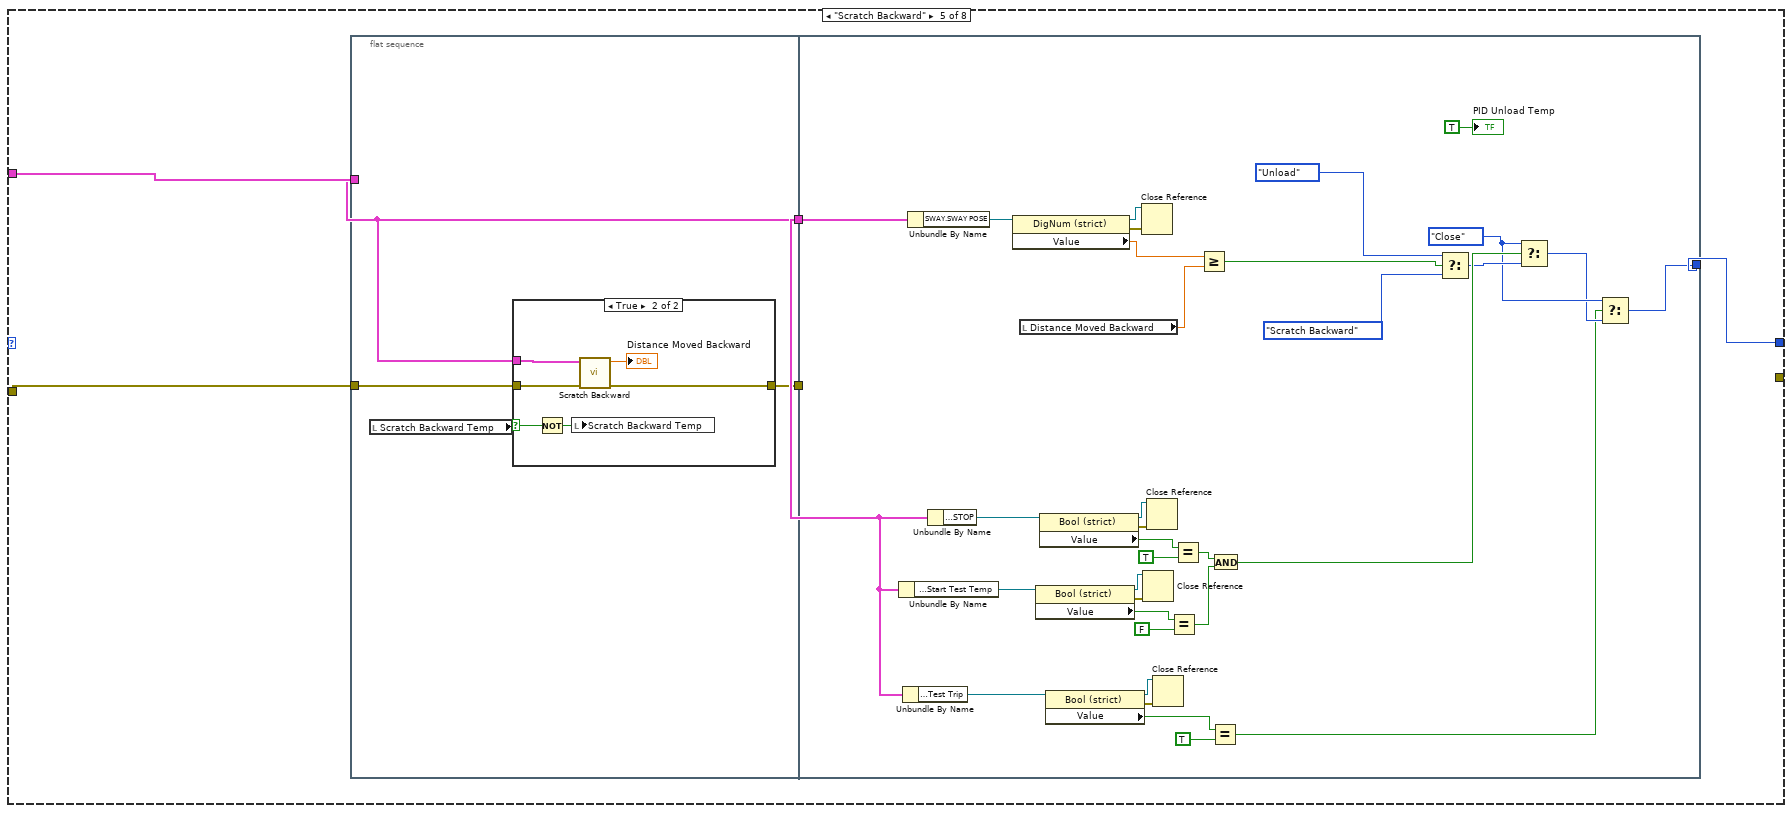
[diagram p15: hidden frame]
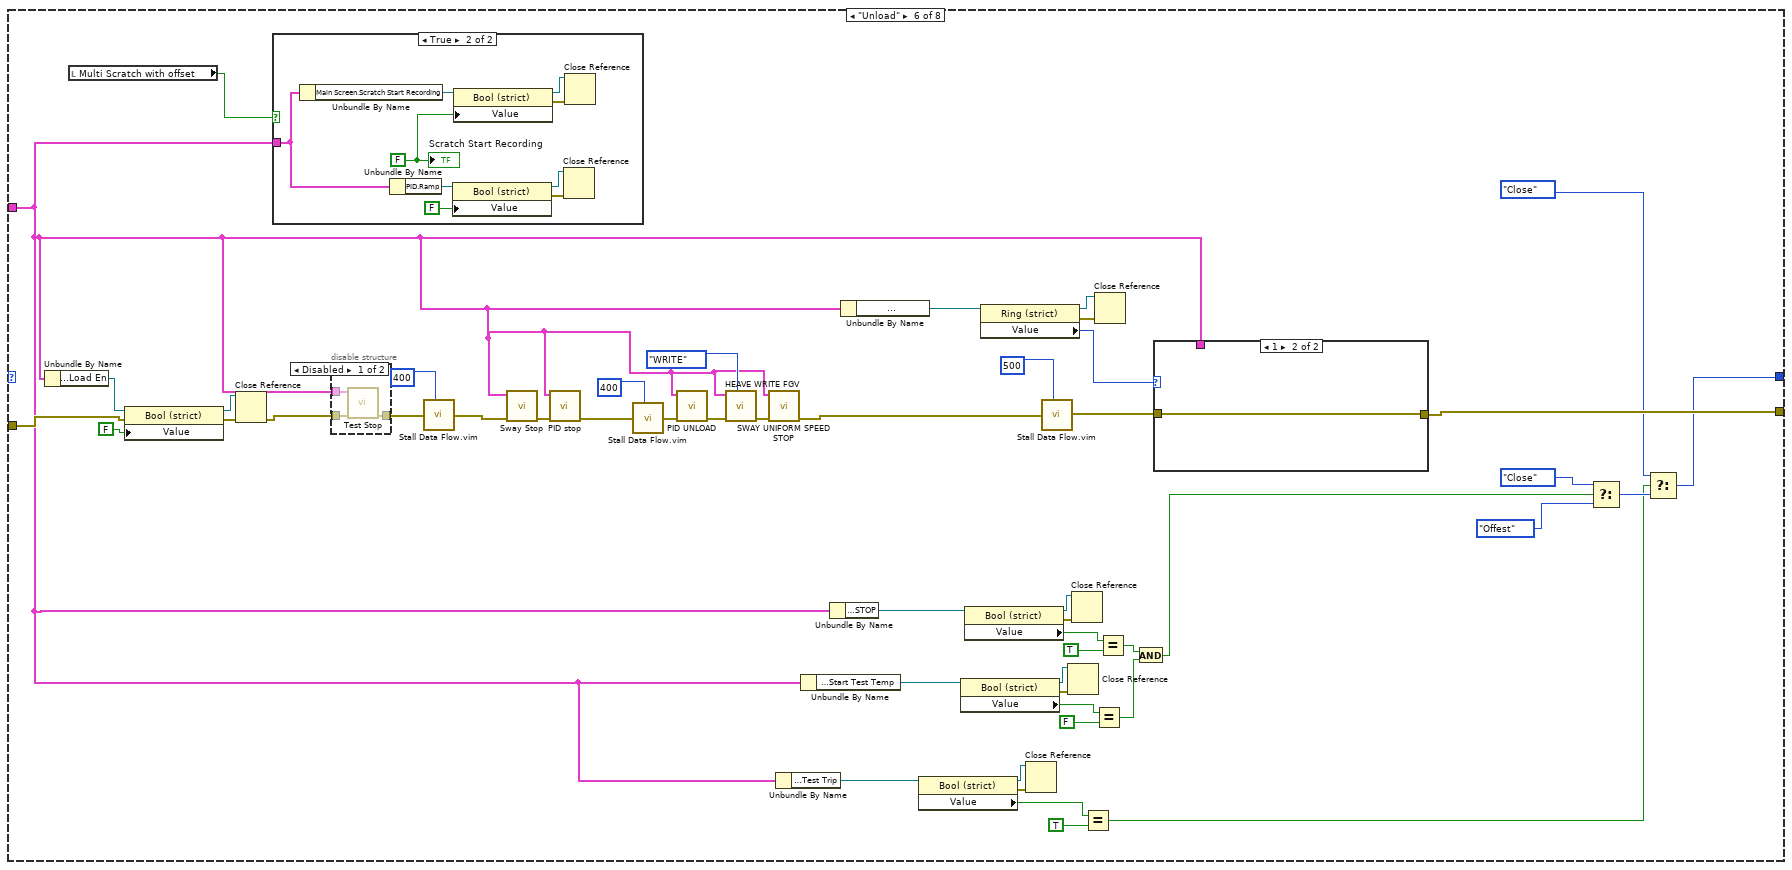
[diagram p17: hidden frame]
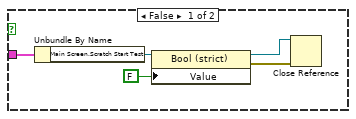
[diagram p18: hidden frame]
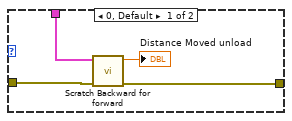
[diagram p20: hidden frame]
diagram:
  # "Init \nLoad\nScratch forward\nScratch Backward\nUnload\nOffset\nclose"
  n1 = case shown="No Error" "error in (no error)" {
    selector: "error in (no error)" -> [w21 _]
    tunnel: "main ref" -> [w4 _]
    frame No Error {
      n2 = Unbundle By Name(w4) -> ("Motion Module.Scratch"=w8:refnum<vi>)
      n3 = Unbundle By Name(w4) -> ("Main Home Screen.GUI"=w18:refnum<vi>)
      n4 = Unbundle By Name(w4) -> ("Main Screen.Start Test Temp"=w13:refnum<vi>)
      n5 = property class="Bool (strict)"(reference=w8) -> (reference out=w5:refnum<vi>, error out=w7:errorcluster, "Value"=w6:bool)  [unwired: 1 in]
      n6 = property class="TabCtl (strict)"(reference=w18) -> (reference out=w20:refnum<vi>, error out=w19:errorcluster, "Value"=w17:T2)  [unwired: 1 in]
      n7 = property class="Bool (strict)"(reference=w13) -> (reference out=w11:refnum<vi>, error out=w12:errorcluster, "Value"=w14:bool)  [unwired: 1 in]
      n8 = Close Reference(reference=w11, error in (no error)=w12) -> ()  [unwired: 1 out]
      n9 = Close Reference(reference=w5, error in (no error)=w7) -> ()  [unwired: 1 out]
      n10 = Equal?(x=w14, y=TRUE) -> (x = y?=w10:bool)
      n11 = Close Reference(reference=w20, error in (no error)=w19) -> ()  [unwired: 1 out]
      n12 = Equal?(x=w17, y=T2."Begin" ("Value")) -> (x = y?=w15:bool)
      n13 = Compound Arithmetic op=AND(w15, w10, w6) -> (w3:bool)
      n14 = case shown="True" w3 {
        tunnel: w4 -> [w23 w78]
        tunnel: w21 -> [_ w77]
        frame False {
          w22 = 0.0 ("Multi Pass Count")
          n15 = Unbundle By Name(w23) -> ("Loading.Loading Mode"=w30:refnum<vi>)
          n16 = property class="Ring (strict)"(reference=w30) -> (reference out=w28:refnum<vi>, error out=w29:errorcluster, "Value"=w27:u16)  [unwired: 1 in]
          n17 = Close Reference(reference=w28, error in (no error)=w29) -> ()  [unwired: 1 out]
          n18 = case shown="0, Default" w27 {
            tunnel: w23 -> [w33 _]
            frame 0, Default {
              n19 = Unbundle By Name(w33) -> ("Motion Module.Scratch"=w51:refnum<vi>)
              n20 = Unbundle By Name(w33) -> ("Motion Module.Enter Scratch Speed (mm/s):"=w46:refnum<vi>)
              n21 = Unbundle By Name(w33) -> ("Motion Module.No of Scratch"=w35:refnum<vi>)
              n22 = Unbundle By Name(w33) -> ("Motion Module.Enter Scratch length (mm):"=w47:refnum<vi>)
              n23 = Unbundle By Name(w33) -> ("Motion Module.Scratch Mode"=w39:refnum<vi>)
              n24 = property class="Bool (strict)"(reference=w51) -> (reference out=w53:refnum<vi>, error out=w52:errorcluster, "Value"=w50:bool)  [unwired: 1 in]
              n25 = property class="DigNum (strict)"(reference=w35) -> (reference out=w34:refnum<vi>, error out=w36:errorcluster, "Value"=w32:dbl)  [unwired: 1 in]
              n26 = property class="Ring (strict)"(reference=w39) -> (reference out=w40:refnum<vi>, error out=w38:errorcluster, "Value"=w37:u16)  [unwired: 1 in]
              n27 = property class="DigNum (strict)"(reference=w47) -> (reference out=w49:refnum<vi>, error out=w48:errorcluster, "Value"=w43:dbl)  [unwired: 1 in]
              n28 = property class="DigNum (strict)"(reference=w46) -> (reference out=w44:refnum<vi>, error out=w45:errorcluster, "Value"=w42:dbl)  [unwired: 1 in]
              n29 = Close Reference(reference=w53, error in (no error)=w52) -> ()  [unwired: 1 out]
              n30 = Close Reference(reference=w34, error in (no error)=w36) -> ()  [unwired: 1 out]
              n31 = Close Reference(reference=w40, error in (no error)=w38) -> ()  [unwired: 1 out]
              n32 = Close Reference(reference=w49, error in (no error)=w48) -> ()  [unwired: 1 out]
              n33 = Close Reference(reference=w44, error in (no error)=w45) -> ()  [unwired: 1 out]
              n34 = case shown="0, Default" w37 {
                tunnel: [1.0 w55] -> w31
                tunnel: w32 -> [_ w55]
                frame 0, Default {
                }
                frame 2 {
                }
              }
              n35 = Divide(x=w43, y=w42) -> (x/y=w41:dbl)
              n36 = case shown="True" w50 {
                tunnel: w33 -> [_ w57]
                tunnel: w41 -> [_ w58]
                tunnel: w31 -> [_ w56]
                frame False {
                }
                frame True {
                  n37 = Unbundle By Name(w57) -> ("Motion Module.Motion type:"=w61:refnum<vi>)
                  n38 = property class="Ring (strict)"(reference=w61) -> (reference out=w62:refnum<vi>, error out=w60:errorcluster, "Value"=w59:u16)  [unwired: 1 in]
                  n39 = Close Reference(reference=w62, error in (no error)=w60) -> ()  [unwired: 1 out]
                  n40 = case shown="0, Default" w59 {
                    tunnel: w58 -> [w64 w72]
                    tunnel: w57 -> [w66 w73]
                    tunnel: w56 -> [w63 _]
                    frame 0, Default {
                      n41 = Unbundle By Name(w66) -> ("Main Screen.Test Duration"=w68:refnum<vi>)
                      n42 = Multiply(x=w64, y=w63) -> (x*y=w65:dbl)
                      n43 = property class="DigNum (strict)"(reference=w68, "Value"=w65) -> (reference out=w69:refnum<vi>, error out=w67:errorcluster)  [unwired: 1 in]
                      n44 = Close Reference(reference=w69, error in (no error)=w67) -> ()  [unwired: 1 out]
                    }
                    frame 1 {
                      n45 = Multiply(x=2.0, y=w72) -> (x*y=w71:dbl)
                      n46 = Unbundle By Name(w73) -> ("Main Screen.Test Duration"=w75:refnum<vi>)
                      n47 = property class="DigNum (strict)"(reference=w75, "Value"=w71) -> (reference out=w76:refnum<vi>, error out=w74:errorcluster)  [unwired: 1 in]
                      n48 = Close Reference(reference=w76, error in (no error)=w74) -> ()  [unwired: 1 out]
                    }
                  }
                }
              }
            }
            frame 1 {
            }
          }
          n49 = local write "Multi Pass Count"(w22) -> ()
          n50 = Unbundle By Name(w23) -> ("Main Screen.Multi Scratch Pass"=w26:refnum<vi>)
          n51 = property class="DigNum (strict)"(reference=w26, "Value"=w22) -> (reference out=w24:refnum<vi>, error out=w25:errorcluster)  [unwired: 1 in]
          n52 = Close Reference(reference=w24, error in (no error)=w25) -> ()  [unwired: 1 out]
        }
        frame True {
          n53 = while {
            shift-right: [w84] -> _
            shift-left: Scratch_Main_Enum."Init" -> [w86]
            tunnel: w78 -> [w85]
            tunnel: w77 -> [w83]
            tunnel: [w81] -> _
            stop <- w80 stop-if-true
            n54 = case shown="\"Close\"" w86 {
              tunnel: w85 -> [w87 w139 w180 w219 w292 w344 w414 w496]
              tunnel: [w99 w141 w176 w215 w288 w338 w418 Scratch_Main_Enum."Init"] -> w84
              tunnel: w83 -> [w112 w165 _ w218 w291 w350 w447 w504]
              tunnel: [w112 w165 _ _ _ w382 w442 w502] -> w81
              tunnel: [_ _ _ _ _ _ _ TRUE] -> w80
              frame "Init", Default {
                n55 = Unbundle By Name(w87) -> ("Motion Module.Scratch Mode"=w97:refnum<vi>)
                n56 = Unbundle By Name(w87) -> ("Main Screen.Start Test Temp"=w135:refnum<vi>)
                n57 = Unbundle By Name(w87) -> ("Main Screen.Start Test"=w132:refnum<vi>)
                n58 = property class="Ring (strict)"(reference=w97) -> (reference out=w98:refnum<vi>, error out=w96:errorcluster, "Value"=w95:u16)  [unwired: 1 in]
                n59 = property class="Bool (strict)"(reference=w135) -> (reference out=w136:refnum<vi>, error out=w134:errorcluster, "Value"=w130:bool)  [unwired: 1 in]
                n60 = Close Reference(reference=w98, error in (no error)=w96) -> ()  [unwired: 1 out]
                n61 = Equal?(x=w95, y=u16 2) -> (x = y?=→"Multi Scratch with offset":bool)
                n62 = property class="Bool (strict)"(reference=w132) -> (reference out=w131:refnum<vi>, error out=w133:errorcluster, "Value"=w129:bool)  [unwired: 1 in]
                n63 = Close Reference(reference=w136, error in (no error)=w134) -> ()  [unwired: 1 out]
                n64 = Close Reference(reference=w131, error in (no error)=w133) -> ()  [unwired: 1 out]
                n65 = And(x=w130, y=w129) -> (x .and. y?=w128:bool)
                n66 = Unbundle By Name(w87) -> ("Main Screen.Start Test Temp"=w122:refnum<vi>)
                n67 = Unbundle By Name(w87) -> ("Main Screen.STOP"=w125:refnum<vi>)
                n68 = Unbundle By Name(w87) -> ("Main Screen.Scratch Start Recording"=w90:refnum<vi>)
                n69 = Unbundle By Name(w87) -> ("Main Screen.Test Trip"=w105:refnum<vi>)
                n70 = Unbundle By Name(w87) -> ("Main Screen.Scratch Start Test"=w110:refnum<vi>)
                n71 = property class="Bool (strict)"(reference=w110, "Value"=FALSE) -> (reference out=w111:refnum<vi>, error out=w109:errorcluster)  [unwired: 1 in]
                n72 = property class="Bool (strict)"(reference=w122) -> (reference out=w120:refnum<vi>, error out=w121:errorcluster, "Value"=w123:bool)  [unwired: 1 in]
                n73 = property class="Bool (strict)"(reference=w125) -> (reference out=w127:refnum<vi>, error out=w126:errorcluster, "Value"=w124:bool)  [unwired: 1 in]
                n74 = property class="Bool (strict)"(reference=w90, "Value"=TRUE) -> (reference out=w91:refnum<vi>, error out=w89:errorcluster)  [unwired: 1 in]
                n75 = property class="Bool (strict)"(reference=w105) -> (reference out=w107:refnum<vi>, error out=w106:errorcluster, "Value"=w103:bool)  [unwired: 1 in]
                n76 = Close Reference(reference=w107, error in (no error)=w106) -> ()  [unwired: 1 out]
                n77 = Close Reference(reference=w111, error in (no error)=w109) -> ()  [unwired: 1 out]
                n78 = Close Reference(reference=w91, error in (no error)=w89) -> ()  [unwired: 1 out]
                n79 = Close Reference(reference=w120, error in (no error)=w121) -> ()  [unwired: 1 out]
                n80 = Close Reference(reference=w127, error in (no error)=w126) -> ()  [unwired: 1 out]
                n81 = Equal?(x=w123, y=FALSE) -> (x = y?=w118:bool)
                n82 = Equal?(x=w124, y=TRUE) -> (x = y?=w119:bool)
                n83 = Equal?(x=w103, y=TRUE) -> (x = y?=w102:bool)
                n84 = And(x=w119, y=w118) -> (x .and. y?=w115:bool)
                n85 = Select(t=Scratch_Main_Enum."Start", s=w128, f=Scratch_Main_Enum."Init") -> (s? t:f=w113:T3)
                n86 = Select(t=Scratch_Main_Enum."Close", s=w115, f=w113) -> (s? t:f=w100:T3)
                n87 = Select(t=Scratch_Main_Enum."Close", s=w102, f=w100) -> (s? t:f=w99:T3)
                "Multi Pass Count" <- 0.0 ("Multi Pass Count")
              }
              frame "Start" {
                n88 = Unbundle By Name(w139) -> ("Main Screen.Load En"=w169:refnum<vi>)
                n89 = property class="Bool (strict)"(reference=w169, "Value"=TRUE) -> (reference out=w167:refnum<vi>, error out=w168:errorcluster)  [unwired: 1 in]
                n90 = Close Reference(reference=w167, error in (no error)=w168) -> ()  [unwired: 1 out]
                n91 = local read "Multi Scratch with offset"() -> (w140:bool)
                n92 = case shown="True" w140 {
                  tunnel: w139 -> [_ w172]
                  frame False {
                  }
                  frame True {
                    n93 = local read "Multi Pass Count"() -> (w171:dbl)
                    n94 = Unbundle By Name(w172) -> ("Main Screen.Multi Scratch Pass"=w175:refnum<vi>)
                    n95 = Increment(x=w171) -> (x+1=w170:dbl)
                    n96 = property class="DigNum (strict)"(reference=w175, "Value"=w170) -> (reference out=w173:refnum<vi>, error out=w174:errorcluster)  [unwired: 1 in]
                    n97 = Close Reference(reference=w173, error in (no error)=w174) -> ()  [unwired: 1 out]
                  }
                }
                n98 = Unbundle By Name(w139) -> ("Main Screen.Start Test Temp"=w159:refnum<vi>)
                n99 = Unbundle By Name(w139) -> ("Main Screen.Test Trip"=w147:refnum<vi>)
                n100 = Unbundle By Name(w139) -> ("Main Screen.STOP"=w162:refnum<vi>)
                n101 = property class="Bool (strict)"(reference=w159) -> (reference out=w157:refnum<vi>, error out=w158:errorcluster, "Value"=w160:bool)  [unwired: 1 in]
                n102 = property class="Bool (strict)"(reference=w162) -> (reference out=w164:refnum<vi>, error out=w163:errorcluster, "Value"=w161:bool)  [unwired: 1 in]
                n103 = property class="Bool (strict)"(reference=w147) -> (reference out=w149:refnum<vi>, error out=w148:errorcluster, "Value"=w145:bool)  [unwired: 1 in]
                n104 = Close Reference(reference=w157, error in (no error)=w158) -> ()  [unwired: 1 out]
                n105 = Close Reference(reference=w164, error in (no error)=w163) -> ()  [unwired: 1 out]
                n106 = Equal?(x=w160, y=FALSE) -> (x = y?=w155:bool)
                n107 = Equal?(x=w161, y=TRUE) -> (x = y?=w156:bool)
                n108 = Close Reference(reference=w149, error in (no error)=w148) -> ()  [unwired: 1 out]
                n109 = And(x=w156, y=w155) -> (x .and. y?=w151:bool)
                n110 = Equal?(x=w145, y=TRUE) -> (x = y?=w143:bool)
                n111 = Select(t=Scratch_Main_Enum."Close", s=w151, f=Scratch_Main_Enum."Load") -> (s? t:f=w142:T3)
                n112 = Select(t=Scratch_Main_Enum."Close", s=w143, f=w142) -> (s? t:f=w141:T3)
              }
              frame "Load" {
                n113 = Unbundle By Name(w180) -> ("Main Screen.NL disp 2"=w214:refnum<vi>)
                n114 = Unbundle By Name(w180) -> ("Main Screen.Set Load (N)"=w210:refnum<vi>)
                n115 = property class="DigNum (strict)"(reference=w214) -> (reference out=w212:refnum<vi>, error out=w213:errorcluster, "Value"=w205:dbl)  [unwired: 1 in]
                n116 = property class="DigNum (strict)"(reference=w210) -> (reference out=w209:refnum<vi>, error out=w211:errorcluster, "Value"=w208:dbl)  [unwired: 1 in]
                n117 = Close Reference(reference=w212, error in (no error)=w213) -> ()  [unwired: 1 out]
                n118 = Close Reference(reference=w209, error in (no error)=w211) -> ()  [unwired: 1 out]
                n119 = Subtract(x=w208, y=0.5) -> (x-y=w206:dbl)
                n120 = Greater Or Equal?(x=w205, y=w206) -> (x >= y?=w202:bool)
                n121 = Unbundle By Name(w180) -> ("Main Screen.Start Test Temp"=w194:refnum<vi>)
                n122 = Unbundle By Name(w180) -> ("Main Screen.Test Trip"=w183:refnum<vi>)
                n123 = Unbundle By Name(w180) -> ("Main Screen.STOP"=w197:refnum<vi>)
                n124 = property class="Bool (strict)"(reference=w194) -> (reference out=w192:refnum<vi>, error out=w193:errorcluster, "Value"=w195:bool)  [unwired: 1 in]
                n125 = property class="Bool (strict)"(reference=w197) -> (reference out=w199:refnum<vi>, error out=w198:errorcluster, "Value"=w196:bool)  [unwired: 1 in]
                n126 = property class="Bool (strict)"(reference=w183) -> (reference out=w185:refnum<vi>, error out=w184:errorcluster, "Value"=w181:bool)  [unwired: 1 in]
                n127 = Close Reference(reference=w192, error in (no error)=w193) -> ()  [unwired: 1 out]
                n128 = Close Reference(reference=w199, error in (no error)=w198) -> ()  [unwired: 1 out]
                n129 = Close Reference(reference=w185, error in (no error)=w184) -> ()  [unwired: 1 out]
                n130 = Equal?(x=w195, y=FALSE) -> (x = y?=w190:bool)
                n131 = Equal?(x=w196, y=TRUE) -> (x = y?=w191:bool)
                n132 = Equal?(x=w181, y=TRUE) -> (x = y?=w179:bool)
                n133 = And(x=w191, y=w190) -> (x .and. y?=w187:bool)
                n134 = Select(t=Scratch_Main_Enum."Scratch Forward", s=w202, f=Scratch_Main_Enum."Load") -> (s? t:f=w186:T3)
                n135 = Select(t=Scratch_Main_Enum."Close", s=w187, f=w186) -> (s? t:f=w178:T3)
                n136 = Select(t=Scratch_Main_Enum."Close", s=w179, f=w178) -> (s? t:f=w176:T3)
                "Scratch Forward Temp" <- TRUE ("Scratch Forward Temp")
              }
              frame "Scratch Forward" {
                n137 = flat-sequence {
                  tunnel: w219 -> [w221]
                  tunnel: w218 -> [w229]
                  tunnel: [w228] -> w217
                  tunnel: [w221] -> w216
                  tunnel: w217 -> [_]
                  tunnel: w216 -> [w251]
                  tunnel: [w247] -> w215
                  frame #0 {
                    w220 = TRUE ("Value")
                    n138 = local read "Scratch Forward Temp"() -> (w230:bool)
                    n139 = Unbundle By Name(w221) -> ("Main Screen.Scratch Start Recording"=w223:refnum<vi>)
                    n140 = case shown="True" w230 {
                      selector: w230 -> [_ w241]
                      tunnel: w221 -> [_ w232]
                      tunnel: w229 -> [w231 w239]
                      tunnel: [w231 w238] -> w228
                      frame False {
                      }
                      frame True {
                        n141 = Unbundle By Name(w232) -> ("Loading.Loading Mode"=w236:refnum<vi>)
                        n142 = property class="Ring (strict)"(reference=w236) -> (reference out=w234:refnum<vi>, error out=w235:errorcluster, "Value"=w233:u16)  [unwired: 1 in]
                        n143 = Not(x=w241) -> (.not. x?=w240:bool)
                        n144 = local write "Scratch Forward Temp"(w240) -> ()
                        n145 = call "Scratch Forward.vi"("error in (no error)"=w239, "main ref"=w232) -> ("error out"=w238:errorcluster, "Distance Moved"=→"Distance Moved":dbl)  [unwired: 8 in]
                        n146 = Close Reference(reference=w234, error in (no error)=w235) -> ()  [unwired: 1 out]
                        n147 = case shown="1" w233 {
                          tunnel: w232 -> [_ w243]
                          frame 0, Default {
                          }
                          frame 1 {
                            n148 = Unbundle By Name(w243) -> ("PID.Ramp"=w244:refnum<vi>)
                            n149 = property class="Bool (strict)"(reference=w244, "Value"=TRUE) -> (reference out=w246:refnum<vi>, error out=w245:errorcluster)  [unwired: 1 in]
                            n150 = Close Reference(reference=w246, error in (no error)=w245) -> ()  [unwired: 1 out]
                          }
                        }
                      }
                    }
                    n151 = Unbundle By Name(w221) -> ("Main Screen.Scratch Start Test"=w226:refnum<vi>)
                    n152 = property class="Bool (strict)"(reference=w223, "Value"=w220) -> (reference out=w224:refnum<vi>, error out=w222:errorcluster)  [unwired: 1 in]
                    n153 = property class="Bool (strict)"(reference=w226, "Value"=w220) -> (reference out=w227:refnum<vi>, error out=w225:errorcluster)  [unwired: 1 in]
                    n154 = local write "Scratch Start Recording"(w220) -> ()
                    n155 = Close Reference(reference=w224, error in (no error)=w222) -> ()  [unwired: 1 out]
                    n156 = Close Reference(reference=w227, error in (no error)=w225) -> ()  [unwired: 1 out]
                  }
                  frame #1 {
                    n157 = Unbundle By Name(w251) -> ("Motion Module.Motion type:"=w276:refnum<vi>)
                    n158 = Unbundle By Name(w251) -> ("Main Screen.Start Test Temp"=w265:refnum<vi>)
                    n159 = Unbundle By Name(w251) -> ("SWAY.SWAY POSE"=w282:refnum<vi>)
                    n160 = Unbundle By Name(w251) -> ("Main Screen.Test Trip"=w254:refnum<vi>)
                    n161 = Unbundle By Name(w251) -> ("Main Screen.STOP"=w268:refnum<vi>)
                    n162 = property class="DigNum (strict)"(reference=w282) -> (reference out=w281:refnum<vi>, error out=w283:errorcluster, "Value"=w280:sgl)  [unwired: 1 in]
                    n163 = property class="Ring (strict)"(reference=w276) -> (reference out=w277:refnum<vi>, error out=w275:errorcluster, "Value"=w274:u16)  [unwired: 1 in]
                    n164 = local read "Distance Moved"() -> (w279:dbl)
                    n165 = property class="Bool (strict)"(reference=w265) -> (reference out=w263:refnum<vi>, error out=w264:errorcluster, "Value"=w266:bool)  [unwired: 1 in]
                    n166 = property class="Bool (strict)"(reference=w268) -> (reference out=w270:refnum<vi>, error out=w269:errorcluster, "Value"=w267:bool)  [unwired: 1 in]
                    n167 = property class="Bool (strict)"(reference=w254) -> (reference out=w256:refnum<vi>, error out=w255:errorcluster, "Value"=w252:bool)  [unwired: 1 in]
                    n168 = Close Reference(reference=w277, error in (no error)=w275) -> ()  [unwired: 1 out]
                    n169 = Close Reference(reference=w281, error in (no error)=w283) -> ()  [unwired: 1 out]
                    n170 = Close Reference(reference=w263, error in (no error)=w264) -> ()  [unwired: 1 out]
                    n171 = Close Reference(reference=w270, error in (no error)=w269) -> ()  [unwired: 1 out]
                    n172 = Equal?(x=w266, y=FALSE) -> (x = y?=w261:bool)
                    n173 = Close Reference(reference=w256, error in (no error)=w255) -> ()  [unwired: 1 out]
                    n174 = Equal?(x=w267, y=TRUE) -> (x = y?=w262:bool)
                    n175 = Less Or Equal?(x=w280, y=w279) -> (x <= y?=w278:bool)
                    n176 = case shown="0, Default" w274 {
                      tunnel: [Scratch_Main_Enum."Unload" Scratch_Main_Enum."Scratch Backward"] -> w273
                      frame 0, Default {
                        n177 = local write "PID Unload Temp"(TRUE ("PID Unload Temp")) -> ()
                      }
                      frame 1 {
                        "Scratch Backward Temp" <- TRUE
                      }
                    }
                    n178 = And(x=w262, y=w261) -> (x .and. y?=w258:bool)
                    n179 = Equal?(x=w252, y=TRUE) -> (x = y?=w249:bool)
                    n180 = Select(t=w273, s=w278, f=Scratch_Main_Enum."Scratch Forward") -> (s? t:f=w257:T3)
                    n181 = Select(t=Scratch_Main_Enum."Close", s=w258, f=w257) -> (s? t:f=w248:T3)
                    n182 = Select(t=Scratch_Main_Enum."Close", s=w249, f=w248) -> (s? t:f=w247:T3)
                  }
                }
              }
              frame "Scratch Backward" {
                n183 = flat-sequence {
                  tunnel: w292 -> [w294]
                  tunnel: w291 -> [w296]
                  tunnel: [w295] -> w290
                  tunnel: [w294] -> w289
                  tunnel: w290 -> [_]
                  tunnel: w289 -> [w308]
                  tunnel: [w305] -> w288
                  frame #0 {
                    n184 = local read "Scratch Backward Temp"() -> (w293:bool)
                    n185 = case shown="True" w293 {
                      selector: w293 -> [_ w299]
                      tunnel: w294 -> [_ w303]
                      tunnel: w296 -> [w297 w302]
                      tunnel: [w297 w301] -> w295
                      frame False {
                      }
                      frame True {
                        n186 = Not(x=w299) -> (.not. x?=w298:bool)
                        n187 = local write "Scratch Backward Temp"(w298) -> ()
                        n188 = call "Scratch Backward.vi"("error in (no error)"=w302, "main ref"=w303) -> ("error out"=w301:errorcluster, "Distance Moved"=→"Distance Moved Backward":dbl)  [unwired: 8 in]
                      }
                    }
                  }
                  frame #1 {
                    w307 = Scratch_Main_Enum."Close"
                    n189 = Unbundle By Name(w308) -> ("Main Screen.Start Test Temp"=w322:refnum<vi>)
                    n190 = Unbundle By Name(w308) -> ("Main Screen.Test Trip"=w311:refnum<vi>)
                    n191 = Unbundle By Name(w308) -> ("SWAY.SWAY POSE"=w335:refnum<vi>)
                    n192 = Unbundle By Name(w308) -> ("Main Screen.STOP"=w325:refnum<vi>)
                    n193 = property class="DigNum (strict)"(reference=w335) -> (reference out=w334:refnum<vi>, error out=w336:errorcluster, "Value"=w333:sgl)  [unwired: 1 in]
                    n194 = local read "Distance Moved Backward"() -> (w332:dbl)
                    n195 = property class="Bool (strict)"(reference=w322) -> (reference out=w320:refnum<vi>, error out=w321:errorcluster, "Value"=w323:bool)  [unwired: 1 in]
                    n196 = property class="Bool (strict)"(reference=w325) -> (reference out=w327:refnum<vi>, error out=w326:errorcluster, "Value"=w324:bool)  [unwired: 1 in]
                    n197 = property class="Bool (strict)"(reference=w311) -> (reference out=w313:refnum<vi>, error out=w312:errorcluster, "Value"=w309:bool)  [unwired: 1 in]
                    n198 = Close Reference(reference=w334, error in (no error)=w336) -> ()  [unwired: 1 out]
                    n199 = Close Reference(reference=w320, error in (no error)=w321) -> ()  [unwired: 1 out]
                    n200 = Close Reference(reference=w327, error in (no error)=w326) -> ()  [unwired: 1 out]
                    n201 = Close Reference(reference=w313, error in (no error)=w312) -> ()  [unwired: 1 out]
                    n202 = Equal?(x=w323, y=FALSE) -> (x = y?=w318:bool)
                    n203 = Equal?(x=w324, y=TRUE) -> (x = y?=w319:bool)
                    n204 = Greater Or Equal?(x=w333, y=w332) -> (x >= y?=w331:bool)
                    n205 = Equal?(x=w309, y=TRUE) -> (x = y?=w304:bool)
                    n206 = And(x=w319, y=w318) -> (x .and. y?=w315:bool)
                    n207 = Select(t=Scratch_Main_Enum."Unload", s=w331, f=Scratch_Main_Enum."Scratch Backward") -> (s? t:f=w314:T3)
                    n208 = Select(t=w307, s=w315, f=w314) -> (s? t:f=w306:T3)
                    n209 = Select(t=w307, s=w304, f=w306) -> (s? t:f=w305:T3)
                    "PID Unload Temp" <- TRUE ("PID Unload Temp")
                  }
                }
              }
              frame "Unload" {
                n210 = Unbundle By Name(w344) -> ("Main Screen.Load En"=w352:refnum<vi>)
                n211 = local read "Multi Scratch with offset"() -> (w337:bool)
                n212 = property class="Bool (strict)"(reference=w352, error in=w350, "Value"=FALSE) -> (reference out=w354:refnum<vi>, error out=w353:errorcluster)
                n213 = Close Reference(reference=w354, error in (no error)=w353) -> (error out=w351:errorcluster)
                n214 = case shown="True" w337 {
                  tunnel: w344 -> [w387 w393]
                  frame False {
                    n215 = Unbundle By Name(w387) -> ("Main Screen.Scratch Start Test"=w390:refnum<vi>)
                    n216 = property class="Bool (strict)"(reference=w390, "Value"=FALSE) -> (reference out=w391:refnum<vi>, error out=w389:errorcluster)  [unwired: 1 in]
                    n217 = Close Reference(reference=w391, error in (no error)=w389) -> ()  [unwired: 1 out]
                  }
                  frame True {
                    w397 = FALSE ("Scratch Start Recording")
                    n218 = Unbundle By Name(w393) -> ("Main Screen.Scratch Start Recording"=w399:refnum<vi>)
                    n219 = Unbundle By Name(w393) -> ("PID.Ramp"=w394:refnum<vi>)
                    n220 = property class="Bool (strict)"(reference=w394, "Value"=FALSE) -> (reference out=w396:refnum<vi>, error out=w395:errorcluster)  [unwired: 1 in]
                    n221 = property class="Bool (strict)"(reference=w399, "Value"=w397) -> (reference out=w400:refnum<vi>, error out=w398:errorcluster)  [unwired: 1 in]
                    n222 = Close Reference(reference=w396, error in (no error)=w395) -> ()  [unwired: 1 out]
                    n223 = Close Reference(reference=w400, error in (no error)=w398) -> ()  [unwired: 1 out]
                    "Scratch Start Recording" <- w397
                  }
                }
                n224 = disable-structure shown="Disabled" {
                  disable-tunnel: w351 -> [w403 w404]
                  disable-tunnel: [w402 w404] -> w357
                  disable-tunnel: w344 -> [w401 _]
                  frame Disabled {
                    n225 = call "Test Stop.vi"("error in (no error)"=w403, "Data Cluster"=w401) -> ("error out"=w402:errorcluster)  [unwired: 9 in]
                  }
                  frame Enabled {
                  }
                }
                n226 = call "Stall Data Flow.vim"("value in"=w357, "milliseconds to wait"=u32 400) -> ("value out"=w349:errorcluster)  [unwired: 1 out]
                n227 = call "Sway Stop.vi"("error in (no error)"=w349, "main ref"=w344) -> ("error out"=w363:errorcluster)  [unwired: 9 in]
                n228 = call "PID stop.vi"("error in (no error)"=w363, "main ref"=w344) -> ("error out"=w364:errorcluster)  [unwired: 9 in]
                n229 = call "Stall Data Flow.vim"("value in"=w364, "milliseconds to wait"=u32 400) -> ("value out"=w360:errorcluster)  [unwired: 1 out]
                n230 = call "PID UNLOAD.vi"("error in (no error)"=w360, "main ref"=w344) -> ("error out"=w359:errorcluster)  [unwired: 9 in]
                n231 = call "HEAVE WRITE FGV.vi"("Enum - Menu"=Heave_Write_enum."WRITE", "error in (no error)"=w359, "main ref"=w344) -> ("error out"=w362:errorcluster)  [unwired: 8 in]
                n232 = call "SWAY UNIFORM SPEED STOP.vi"("error in (no error)"=w362, "Data Cluster"=w344) -> ("error out"=w356:errorcluster)  [unwired: 9 in]
                n233 = Unbundle By Name(w344) -> ("Main Screen.Test Trip"=w345:refnum<vi>)
                n234 = Unbundle By Name(w344) -> ("Main Screen.Start Test Temp"=w375:refnum<vi>)
                n235 = Unbundle By Name(w344) -> ("Main Screen.STOP"=w378:refnum<vi>)
                n236 = Unbundle By Name(w344) -> ("Motion Module.Motion type:"=w385:refnum<vi>)
                n237 = property class="Bool (strict)"(reference=w345) -> (reference out=w347:refnum<vi>, error out=w346:errorcluster, "Value"=w342:bool)  [unwired: 1 in]
                n238 = property class="Bool (strict)"(reference=w375) -> (reference out=w373:refnum<vi>, error out=w374:errorcluster, "Value"=w376:bool)  [unwired: 1 in]
                n239 = property class="Bool (strict)"(reference=w378) -> (reference out=w380:refnum<vi>, error out=w379:errorcluster, "Value"=w377:bool)  [unwired: 1 in]
                n240 = property class="Ring (strict)"(reference=w385) -> (reference out=w386:refnum<vi>, error out=w384:errorcluster, "Value"=w383:u16)  [unwired: 1 in]
                n241 = Close Reference(reference=w347, error in (no error)=w346) -> ()  [unwired: 1 out]
                n242 = call "Stall Data Flow.vim"("value in"=w356, "milliseconds to wait"=u32 500) -> ("value out"=w366:errorcluster)  [unwired: 1 out]
                n243 = Close Reference(reference=w373, error in (no error)=w374) -> ()  [unwired: 1 out]
                n244 = Close Reference(reference=w380, error in (no error)=w379) -> ()  [unwired: 1 out]
                n245 = Equal?(x=w342, y=TRUE) -> (x = y?=w339:bool)
                n246 = Equal?(x=w376, y=FALSE) -> (x = y?=w371:bool)
                n247 = Close Reference(reference=w386, error in (no error)=w384) -> ()  [unwired: 1 out]
                n248 = Equal?(x=w377, y=TRUE) -> (x = y?=w372:bool)
                n249 = And(x=w372, y=w371) -> (x .and. y?=w368:bool)
                n250 = case shown="1" w383 {
                  tunnel: w366 -> [w408 w409]
                  tunnel: w344 -> [w407 _]
                  tunnel: [w406 w409] -> w382
                  frame 0, Default {
                    n251 = call "Scratch Backward for forward.vi"("error in (no error)"=w408, "main ref"=w407) -> ("error out"=w406:errorcluster, "Distance Moved"=→"Distance Moved unload":dbl)  [unwired: 8 in]
                  }
                  frame 1 {
                  }
                }
                n252 = Select(t=Scratch_Main_Enum."Close", s=w368, f=Scratch_Main_Enum."Offest") -> (s? t:f=w341:T3)
                n253 = Select(t=Scratch_Main_Enum."Close", s=w339, f=w341) -> (s? t:f=w338:T3)
              }
              frame "Offest" {
                n254 = Unbundle By Name(w414) -> ("Motion Module.Motion type:"=w445:refnum<vi>)
                n255 = local read "Multi Pass Count"() -> (w412:dbl)
                n256 = property class="Ring (strict)"(reference=w445) -> (reference out=w446:refnum<vi>, error out=w444:errorcluster, "Value"=w443:u16)  [unwired: 1 in]
                n257 = local read "Multi Scratch with offset"() -> (w413:bool)
                n258 = Unbundle By Name(w414) -> ("Motion Module.No of Scratch"=w416:refnum<vi>)
                n259 = Close Reference(reference=w446, error in (no error)=w444) -> ()  [unwired: 1 out]
                n260 = property class="DigNum (strict)"(reference=w416) -> (reference out=w417:refnum<vi>, error out=w415:errorcluster, "Value"=w411:dbl)  [unwired: 1 in]
                n261 = Greater Or Equal?(x=w412, y=w411) -> (x >= y?=w410:bool)
                n262 = case shown="True" w413 {
                  tunnel: w414 -> [w448 w453]
                  tunnel: w410 -> [_ w454]
                  frame False {
                    n263 = Unbundle By Name(w448) -> ("Main Screen.Scratch Start Test"=w451:refnum<vi>)
                    n264 = property class="Bool (strict)"(reference=w451, "Value"=FALSE) -> (reference out=w452:refnum<vi>, error out=w450:errorcluster)  [unwired: 1 in]
                    n265 = Close Reference(reference=w452, error in (no error)=w450) -> ()  [unwired: 1 out]
                  }
                  frame True {
                    n266 = case shown="True" w454 {
                      tunnel: w453 -> [_ w455]
                      frame False {
                      }
                      frame True {
                        n267 = Unbundle By Name(w455) -> ("Main Screen.Scratch Start Test"=w458:refnum<vi>)
                        n268 = property class="Bool (strict)"(reference=w458, "Value"=FALSE) -> (reference out=w459:refnum<vi>, error out=w457:errorcluster)  [unwired: 1 in]
                        n269 = Close Reference(reference=w459, error in (no error)=w457) -> ()  [unwired: 1 out]
                      }
                    }
                  }
                }
                n270 = case shown="0, Default" w443 {
                  tunnel: w414 -> [w463 w493]
                  tunnel: w447 -> [w466 w492]
                  tunnel: [w461 w491] -> w442
                  tunnel: [w464 Scratch_Main_Enum."Close"] -> w427
                  tunnel: w411 -> [w460 _]
                  frame 0, Default {
                    n271 = Unbundle By Name(w463) -> ("SWAY.SWAY POSE"=w468:refnum<vi>)
                    n272 = local read "Distance Moved unload"() -> (w471:dbl)
                    n273 = property class="DigNum (strict)"(reference=w468, error in=w466) -> (reference out=w469:refnum<vi>, error out=w467:errorcluster, "Value"=w470:sgl)
                    n274 = Greater Or Equal?(x=w470, y=w471) -> (x >= y?=w465:bool)
                    n275 = Close Reference(reference=w469, error in (no error)=w467) -> (error out=w462:errorcluster)
                    n276 = case shown="True" w465 {
                      tunnel: [Scratch_Main_Enum."Offest" w477] -> w464
                      tunnel: w463 -> [_ w480]
                      tunnel: w462 -> [w472 w479]
                      tunnel: [w472 w478] -> w461
                      tunnel: w460 -> [_ w474]
                      frame False {
                      }
                      frame True {
                        n277 = local read "Multi Scratch with offset"() -> (w476:bool)
                        n278 = call "Surge Forward in Scratch.vi"("error in (no error)"=w479, "main ref"=w480) -> ("error out"=w478:errorcluster)  [unwired: 9 in]
                        n279 = local read "Multi Pass Count"() -> (w475:dbl)
                        n280 = case shown="True" w476 {
                          tunnel: [Scratch_Main_Enum."Close" w487] -> w477
                          tunnel: w475 -> [_ w484]
                          tunnel: w474 -> [_ w483]
                          frame False {
                          }
                          frame True {
                            n281 = Decrement(x=w483) -> (x-1=w482:dbl)
                            n282 = Increment(x=w484) -> (x+1=w486:dbl)
                            n283 = Greater Or Equal?(x=w484, y=w482) -> (x >= y?=w485:bool)
                            n284 = local write "Multi Pass Count"(w486) -> ()
                            n285 = case shown="True" w485 {
                              tunnel: [Scratch_Main_Enum."Start" Scratch_Main_Enum."Close"] -> w487
                              frame False {
                              }
                              frame True {
                              }
                            }
                          }
                        }
                      }
                    }
                  }
                  frame 1 {
                    n286 = call "Surge Forward in Scratch.vi"("error in (no error)"=w492, "main ref"=w493) -> ("error out"=w491:errorcluster)  [unwired: 9 in]
                  }
                }
                n287 = Close Reference(reference=w417, error in (no error)=w415) -> ()  [unwired: 1 out]
                n288 = Unbundle By Name(w414) -> ("Main Screen.Start Test Temp"=w435:refnum<vi>)
                n289 = Unbundle By Name(w414) -> ("Main Screen.Test Trip"=w423:refnum<vi>)
                n290 = Unbundle By Name(w414) -> ("Main Screen.STOP"=w438:refnum<vi>)
                n291 = property class="Bool (strict)"(reference=w435) -> (reference out=w433:refnum<vi>, error out=w434:errorcluster, "Value"=w436:bool)  [unwired: 1 in]
                n292 = property class="Bool (strict)"(reference=w438) -> (reference out=w440:refnum<vi>, error out=w439:errorcluster, "Value"=w437:bool)  [unwired: 1 in]
                n293 = property class="Bool (strict)"(reference=w423) -> (reference out=w425:refnum<vi>, error out=w424:errorcluster, "Value"=w421:bool)  [unwired: 1 in]
                n294 = Close Reference(reference=w433, error in (no error)=w434) -> ()  [unwired: 1 out]
                n295 = Close Reference(reference=w440, error in (no error)=w439) -> ()  [unwired: 1 out]
                n296 = Close Reference(reference=w425, error in (no error)=w424) -> ()  [unwired: 1 out]
                n297 = Equal?(x=w436, y=FALSE) -> (x = y?=w431:bool)
                n298 = Equal?(x=w437, y=TRUE) -> (x = y?=w432:bool)
                n299 = Equal?(x=w421, y=TRUE) -> (x = y?=w420:bool)
                n300 = And(x=w432, y=w431) -> (x .and. y?=w428:bool)
                n301 = Select(t=Scratch_Main_Enum."Close", s=w428, f=w427) -> (s? t:f=w419:T3)
                n302 = Select(t=Scratch_Main_Enum."Close", s=w420, f=w419) -> (s? t:f=w418:T3)
              }
              frame "Close" {
                n303 = Unbundle By Name(w496) -> ("Main Screen.Test Trip"=w499:refnum<vi>)
                n304 = property class="Bool (strict)"(reference=w499) -> (reference out=w501:refnum<vi>, error out=w500:errorcluster, "Value"=w497:bool)  [unwired: 1 in]
                n305 = Close Reference(reference=w501, error in (no error)=w500) -> ()  [unwired: 1 out]
                n306 = Equal?(x=w497, y=TRUE) -> (x = y?=w495:bool)
                n307 = local write "Multi Scratch with offset"(FALSE ("Multi Scratch with offset")) -> ()
                n308 = case shown="True" w495 {
                  tunnel: w504 -> [w508 w509]
                  tunnel: [w507 w509] -> w502
                  tunnel: w496 -> [w506 _]
                  frame False {
                    n309 = call "Sway Stop.vi"("error in (no error)"=w508, "main ref"=w506) -> ("error out"=w507:errorcluster)  [unwired: 9 in]
                  }
                  frame True {
                  }
                }
                n310 = case shown="False" w495 {
                  tunnel: w496 -> [w512 _]
                  frame False {
                    n311 = Unbundle By Name(w512) -> ("Loading.Loading Mode"=w526:refnum<vi>)
                    n312 = Unbundle By Name(w512) -> ("Main Screen.Start Test"=w540:refnum<vi>)
                    n313 = Unbundle By Name(w512) -> ("Main Screen.STOP"=w529:refnum<vi>)
                    n314 = Unbundle By Name(w512) -> ("Main Screen.Start Test Temp"=w530:refnum<vi>)
                    n315 = Unbundle By Name(w512) -> ("Main Screen.Load En"=w538:refnum<vi>)
                    n316 = property class="Ring (strict)"(reference=w526) -> (reference out=w524:refnum<vi>, error out=w525:errorcluster, "Value"=w523:u16)  [unwired: 1 in]
                    n317 = Close Reference(reference=w524, error in (no error)=w525) -> ()  [unwired: 1 out]
                    n318 = property class="Bool (strict)"(reference=w529, "Value"=FALSE, "Visible"=TRUE) -> (reference out=w527:refnum<vi>, error out=w528:errorcluster)  [unwired: 1 in]
                    n319 = property class="Bool (strict)"(reference=w530, "Value"=FALSE) -> (reference out=w532:refnum<vi>, error out=w531:errorcluster)  [unwired: 1 in]
                    n320 = property class="Bool (strict)"(reference=w538, "Value"=FALSE) -> (reference out=w536:refnum<vi>, error out=w537:errorcluster)  [unwired: 1 in]
                    n321 = property class="Bool (strict)"(reference=w540, "Value"=FALSE, "Visible"=TRUE) -> (reference out=w542:refnum<vi>, error out=w541:errorcluster)  [unwired: 1 in]
                    n322 = case shown="0, Default" w523 {
                      tunnel: w512 -> [_ w546]
                      frame 0, Default {
                      }
                      frame 1 {
                        n323 = Unbundle By Name(w546) -> ("PID.Ramp"=w547:refnum<vi>)
                        n324 = property class="Bool (strict)"(reference=w547, "Value"=FALSE) -> (reference out=w549:refnum<vi>, error out=w548:errorcluster)  [unwired: 1 in]
                        n325 = Close Reference(reference=w549, error in (no error)=w548) -> ()  [unwired: 1 out]
                      }
                    }
                    n326 = Close Reference(reference=w527, error in (no error)=w528) -> ()  [unwired: 1 out]
                    n327 = Close Reference(reference=w532, error in (no error)=w531) -> ()  [unwired: 1 out]
                    n328 = Close Reference(reference=w536, error in (no error)=w537) -> ()  [unwired: 1 out]
                    n329 = Close Reference(reference=w542, error in (no error)=w541) -> ()  [unwired: 1 out]
                    n330 = Unbundle By Name(w512) -> ("Main Screen.Scratch Start Test"=w521:refnum<vi>)
                    n331 = Unbundle By Name(w512) -> ("Main Screen.Scratch Start Recording"=w514:refnum<vi>)
                    n332 = Unbundle By Name(w512) -> ("Motion Module.Scratch Mode"=w517:refnum<vi>)
                    n333 = property class="Bool (strict)"(reference=w521, "Value"=FALSE) -> (reference out=w522:refnum<vi>, error out=w520:errorcluster)  [unwired: 1 in]
                    n334 = property class="Ring (strict)"(reference=w517, "Value"=u16 0) -> (reference out=w516:refnum<vi>, error out=w518:errorcluster)  [unwired: 1 in]
                    n335 = property class="Bool (strict)"(reference=w514, "Value"=FALSE) -> (reference out=w515:refnum<vi>, error out=w513:errorcluster)  [unwired: 1 in]
                    n336 = Close Reference(reference=w522, error in (no error)=w520) -> ()  [unwired: 1 out]
                    n337 = Close Reference(reference=w516, error in (no error)=w518) -> ()  [unwired: 1 out]
                    n338 = Close Reference(reference=w515, error in (no error)=w513) -> ()  [unwired: 1 out]
                  }
                  frame True {
                  }
                }
              }
            }
            n339 = Wait (ms)(milliseconds to wait=u32 200) -> ()  [unwired: 1 out]
          }
        }
      }
    }
    frame Error {
    }
  }
